vi "D-VASim (Dynamic Virtual Analyzer and Simulator).vi"() -> ()   [LabVIEW 2014]
doc: "D-VASim: Dynamic Virtual Analyzer and Simulator\n\nCreated by Hasan Baig (haba@dtu.dk) at Technical University of Denmark (DTU).s"
uses:
  <vilib>/Utility/miscctls.llb/LVRangeTypeDef.ctl
  <vilib>/Simulation/Implementation/Shared/SIM Continuous Solvers.ctl
  <vilib>/Analysis/Matrix/Datatypes/RealMatrix.ctl
  Sim_Results/SubVIs/Model Information.ctl
  <vilib>/Utility/miscctls.llb/LVPositionTypeDef.ctl
  <vilib>/Utility/error.llb/DialogType.ctl
  Sim_Results/SubVIs/Path.ctl
  <vilib>/Utility/file.llb/Write To Spreadsheet File (string).vi
  <vilib>/Analysis/Matrix/NI_Matrix.lvlib
  <vilib>/Utility/miscctls.llb/LVPointTypeDef.ctl
  <vilib>/Utility/miscctls.llb/LVBoundsTypeDef.ctl
panel:
  out "SBML Components":string
  out "Fn Arg Cnt":string[](array[string])
  out "Comp IDs":string[](array[string])
  out "New Total Pr IDs":string[](array[string])
  out "Math-w/-ch-VarID":string[](array[string])
  out "LP-Cnt_4_Reac":string[](array[string])
  out "Top 3":i32
  out "Top 2":i32
  out "Top 1":i32
  out "Position 10":T1
  out "Position 6":T1
  out "Position 5":T1
  out "Position 4":T1
  out "Left 3":i32
  out "Left 2":i32
  out "Left 1":i32
  out "Position 9":T1
  out "Position 8":T1
  out "Position 7":T1
  out "Position 3":T1
  out "Position 2":T1
  out "Position":T1
  in  "Mod Range":T2={"Minimum"=0.0, "Maximum"=100.0, "Increment"=1.0, "Minor Increment"=1.0, "Start"=0.0}
  in  "Mod_Dimension":u32=62
  out "OnlySubstanceUnits":string[](array[string])
  out "Bound Cond":string[](array[string])
  in  "Final Time":dbl=100.0
  in  "Initial Time":dbl
  in  "ODE Simulation Parameters":T4={"Time Step"=0.1, "Absolute Tolerance"=0.001, "Relative Tolerance"=1e-06, "Continuous Solver"=enum."Adams-Moulton (variable)", "Discrete Time Step"=2.0, "Minimum Time Step"=1e-06, "Maximum Time Step"=1.0, "Initial Time Step"=0.01} {"Initial Time Step" min=0.0; "Maximum Time Step" min=0.0; "Minimum Time Step" min=0.0; "Discrete Time Step" min=0.0; "Relative Tolerance" min=0.0; "Absolute Tolerance" min=0.0; "Time Step" min=0.0}
  out "Pr_Value":string[](array[string])
  out "Pr_Name":string[](array[string])
  out "Pr_Id_Arr":string[](array[string])
  out "Sp_Init_Amnt":string[](array[string])
  out "Sp_Id_Arr":string[](array[string])
  out "Sp_Name":string[](array[string])
  out "Rest_Sp_IDs":string[](array[string])
  out "Rest_Sp_Init_Amnt":string[](array[string])
  out "Rest_Sp_IDs+Names":string[](array[string])
  out "Delta Matrix":T5
  out "Reactant Matrix":T5
  out "Idx of Mod in Sp IDs":i32[](array[numeric])
  out "Out_Tot_Param":string[](array[string])
  out "Out_X_for_ODE":string[](array[string])
  out "Ex_Mod_Init_Amnt":string[](array[string])
  in  "Obtain parameters from Cello UCF":bool
  out "Model Information":T6
  in  "Select SBML Model (.xml)":path
  in  "Generate ODE VI":bool
  in  "Generate SSA VI":bool
  out "Init Sp State (N)":i32[](array[numeric])
  out "Nxt Sp State (N)":i32[](array[numeric])
  out "Equations":string[](array[string])
  out "Sp_for_ODE+Names(X)":string[](array[string])
  out "SP-for-ODE(X)":string[](array[string])
  out "Ex_Mod_IDs":string[](array[string])
  out "ODE File Name":string
  out "ODE VI Name":string
  out "SSA FileName":string
  in  "Tab Control":T7(tab)
  out "Species Info":string[][](table)
  out "Total Species":i32
  out "Parameter info":string[][](table)
  out "Total Parameters":i32
  out "Ordinary Differential Equations":string[][](table)
  out "Reaction Info":string[][](table)
  out "Reaction Math":string[][](table)
  out "Total Reactions":i32
  out "Event Info":string[][](table)
  out "Total Events":i32
  out "Functions Definition":string[][](table)
  out "Total Function Definitions":i32
  out "Units Definition":string[][](table)
  out "Total Units Definitions":i32
  out "Compartments Definition":string[][](table)
  out "Total Compartments":i32
  out "Total Initial Assignments":i32
  out "Initial Assignment":string[][](table)
  out "Rules":string[][](table)
  out "Total Rules":i32
  out "Total Constraints":i32
  out "Constraints":string[][](table)
  out "SSA VI Name":string
  out "Model Folder":path
  out "standard output":string
  out "LP_Values":string[](array[string])
  out "Reactants_Arr":string[](array[string])
  out "Modifiers_Arr":string[](array[string])
  out "LP_IDs":string[](array[string])
  out "Products_Arr":string[](array[string])
  out "R-Stoich":string[](array[string])
  out "P-Stoich":string[](array[string])
  out "Local Parameter Info":string[][](array[string])
  out "standard error":string
  out "Model Name":string
  out "All Param Names":string[](array[string])
  out "All Param Values":string[](array[string])
  out "Init Sp State (S)":string[](array[string])
  out "Nxt Sp State (S)":string[](array[string])
  out "Out_ODE":string[](array[string])
  out "Total Param_IDs":string[](array[string])
  out "Math Expressions":string[](array[string])
  out "SP_for_ODE_Init_Amnt(X)":string[](array[string])
  out "reference Graph":refnum<vi>
  out "Ex_Mod_List":string[](array[string]) caption="Out_List"
  # "D-VASim: Dynamic Virtual Analyzer and Simulator"
  # "Technical University of Denmark"
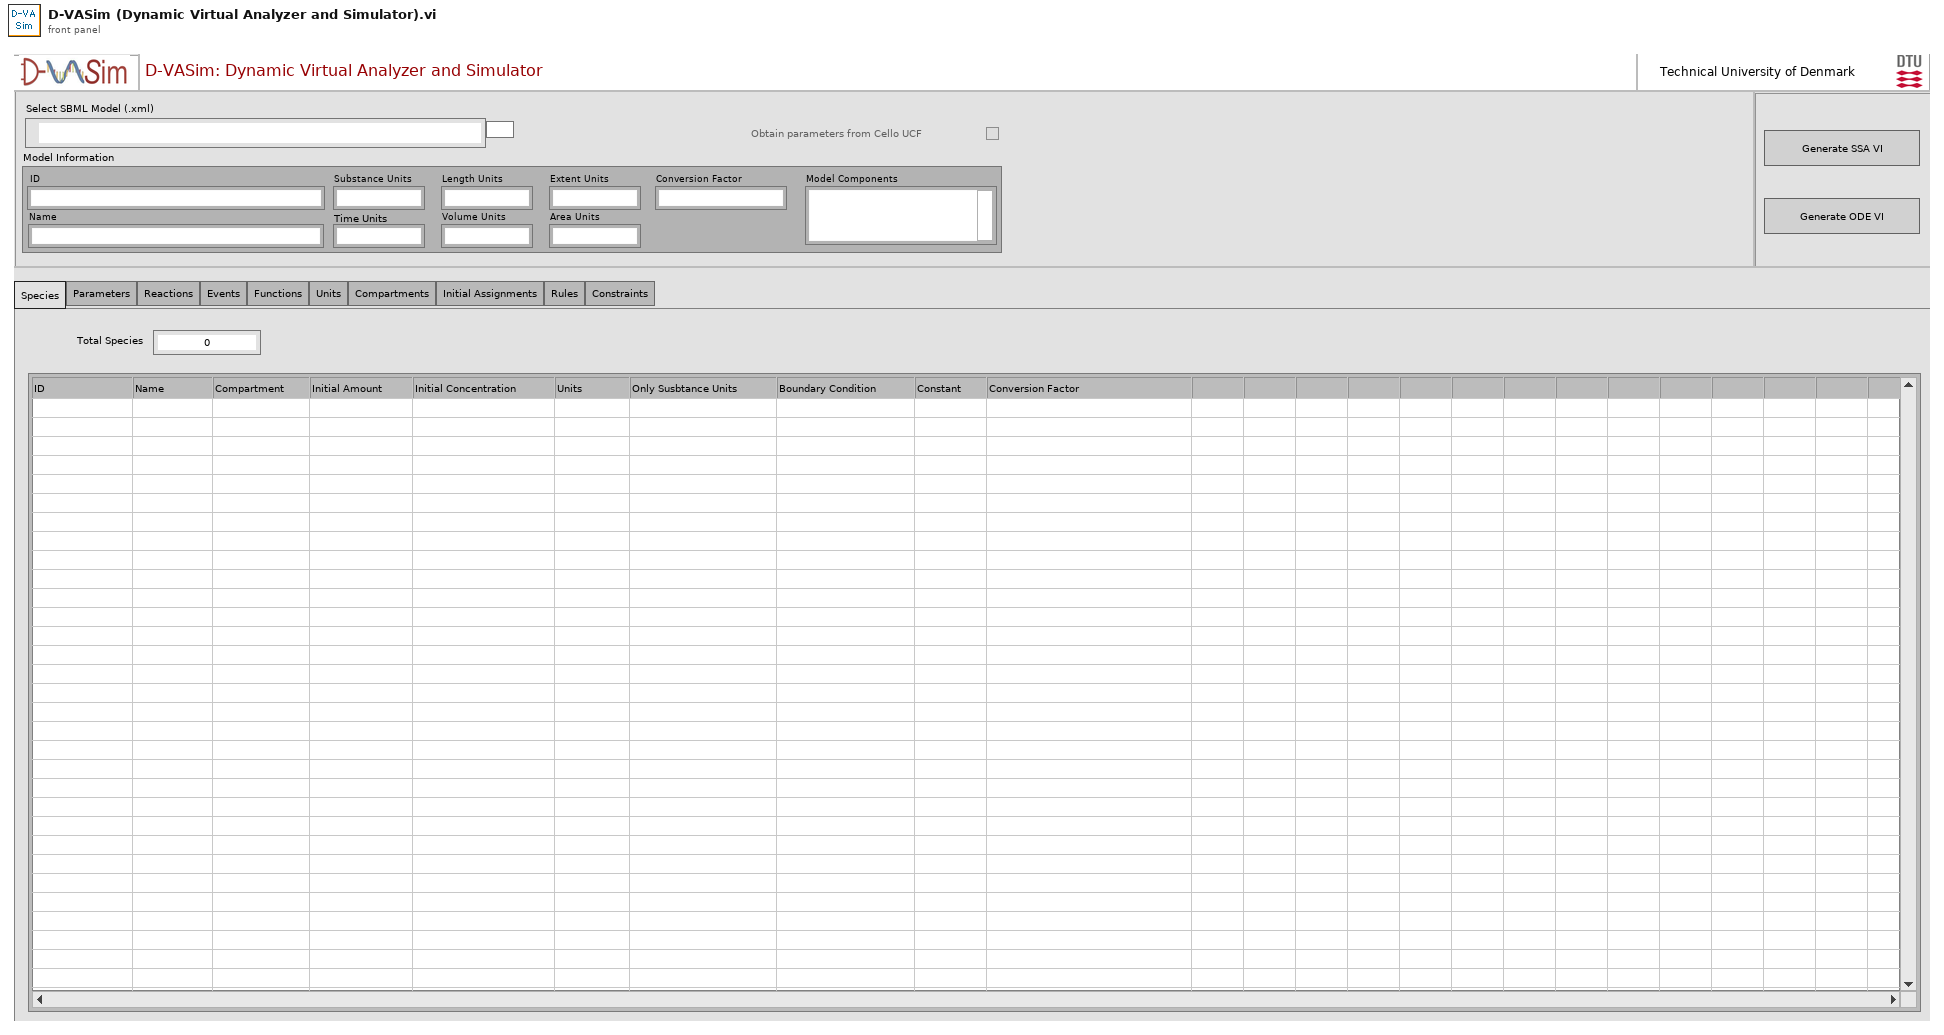
[diagram p1: front panel]
types:
  T1 = typedef "LVPositionTypeDef.ctl" = cluster{"Left":i32, "Top":i32}
  T2 = typedef "LVRangeTypeDef.ctl" = cluster{"Minimum":dbl, "Maximum":dbl, "Increment":dbl, "Minor Increment":dbl, "Start":dbl}
  T3 = typedef "SIM Continuous Solvers.ctl" = enum16{"Runge-Kutta 1 (Euler)", "Runge-Kutta 2", "Runge-Kutta 3", "Runge-Kutta 4", "Runge-Kutta 23 (variable)", "Runge-Kutta 45 (variable)", "BDF (variable)", "Adams-Moulton (variable)", "Rosenbrock (variable)", "Discrete States Only"}
  T4 = cluster{"Time Step":dbl, "Absolute Tolerance":dbl, "Relative Tolerance":dbl, "Continuous Solver":T3, "Discrete Time Step":dbl, "Minimum Time Step":dbl, "Maximum Time Step":dbl, "Initial Time Step":dbl}
  T5 = typedef "NI_Matrix.lvlib/RealMatrix.ctl" = dbl[][]
  T6 = typedef "Model Information.ctl" = cluster{"ID":string, "Name":string, "Substance Units":string, "Time Units":string, "Volume Units":string, "Area Units":string, "Length Units":string, "Extent Units":string, "Conversion Factor":string, "Model Components":string}
  T7 = enum32{"Species", "Parameters", "Reactions", "Events", "Functions", "Units", "Compartments", "Initial Assignments", "Rules", "Constraints"}
  T8 = typedef "DialogType.ctl" = u16
  T9 = typedef "Path.ctl" = string
  T10 = enum32{"Invalid", "Standard", "Closed", "Hidden", "Minimized", "Maximized"}
  T11 = typedef "LVBoundsTypeDef.ctl" = cluster{"Width":u32, "Height":u32}
  T12 = typedef "LVPointTypeDef.ctl" = cluster{"Horizontal":i16, "Vertical":i16}
  T13 = enum32{"invalid app kind", "Development System", "Run Time System", "Student Edition", "Embedded LabVIEW", "Evaluation", "Custom"}
  T14 = cluster{"Model Info":T6, "SpCnt":i32, "Species Info":string[][], "Pr_Cnt":i32, "Parameter info":string[][], "ReacCnt":i32, "Reaction Info":string[][], "Math Expressions":string[][], "EventsCnt":i32, "Event Info":string[][], "UnitsDefCnt":i32, "Units Def":string[][], "CompCnt":i32, "Comp Def":string[][], "Mod_ID":string[], "Mod_Idx":i32[], "RulesCnt":i32, "Rules":string[][], "FuncCnt":i32, "Functions":string[][], "InitAssign Cnt":i32, "Init Assigns":string[][], "ConstraintsCnt":i32, "Constraints":string[][], "Fn Arg Cnt":string[]}
  T15 = cluster{"Reactants_Arr":string[], "R-Stoich":string[], "Products_Arr":string[], "Math Expressions":string[], "P-Stoich":string[], "Bound Cond":string[], "Sp_Id_Arr":string[], "Math-w/-ch-VarID":string[], "OnlySubstanceUnits":string[], "Comp IDs":string[]}
  T16 = cluster{"SP-for-ODE":string[], "Modifiers_Arr":string[], "Sp_Id_Arr":string[], "Sp_Name":string[], "Sp_Init_Amnt":string[], "Reactants_Arr":string[], "Products_Arr":string[]}
  T17 = cluster{"Ex_Mod_IDs":string[], "Ex_Mod_IDs+Names":string[], "Ex_Mod_Init_Amnt":string[], "Rest_Sp_IDs ":string[], "Rest_Sp_IDs+Names":string[], "Rest_Sp_Init_Amnt":string[], "SP_for_ODE_Init_Amnt":string[], "Sp_for_ODE+Names":string[]}
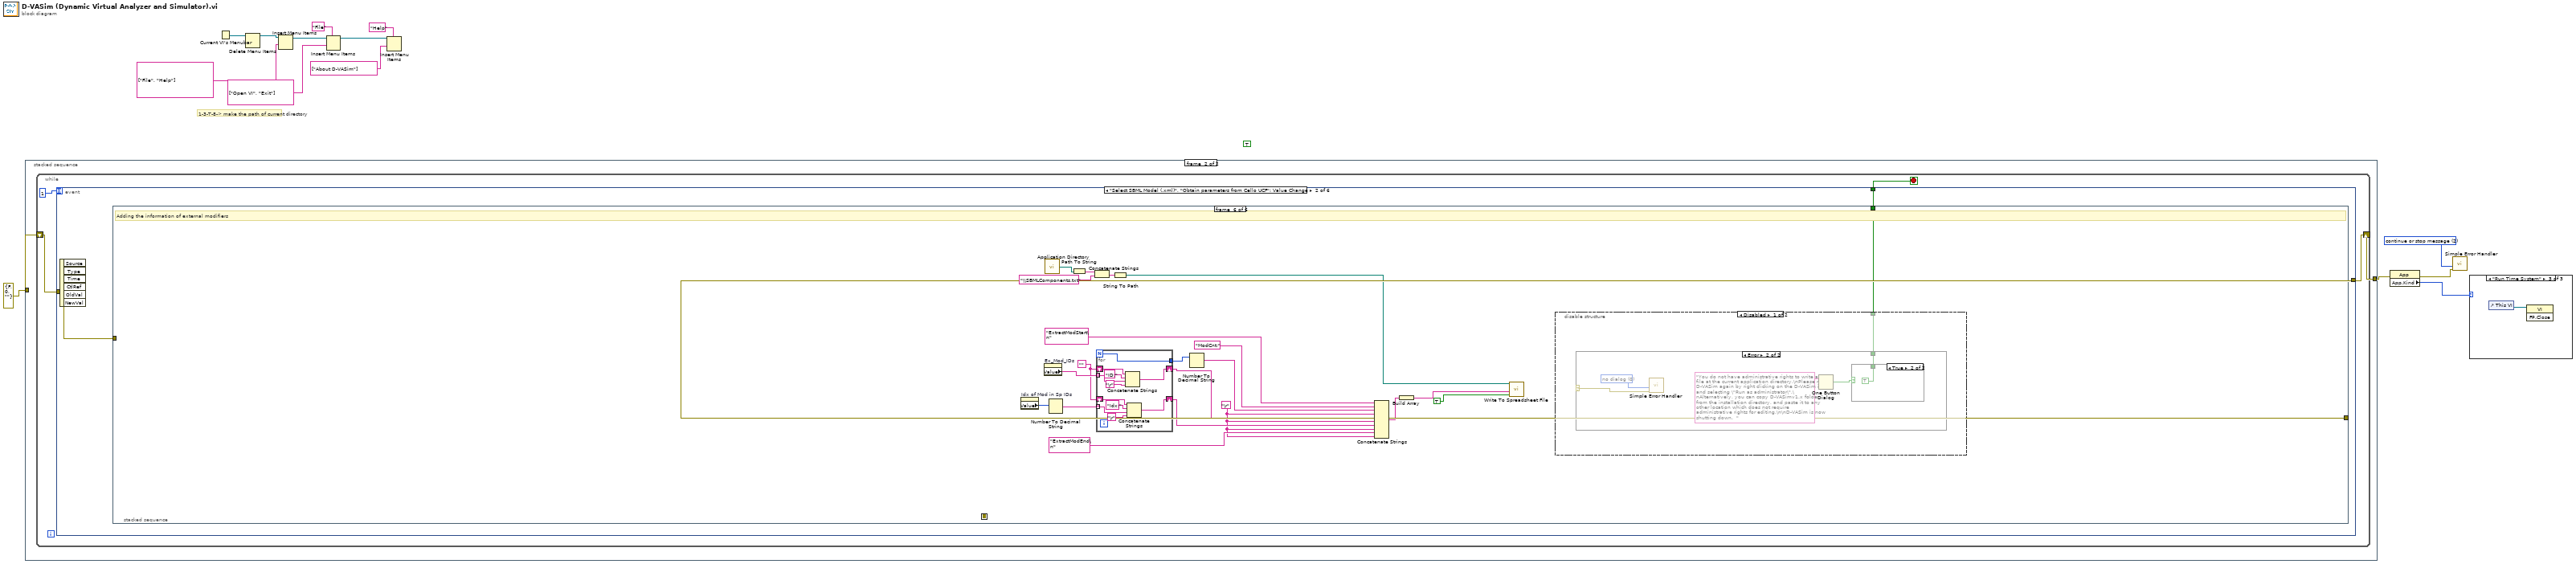
[diagram p0: block diagram]
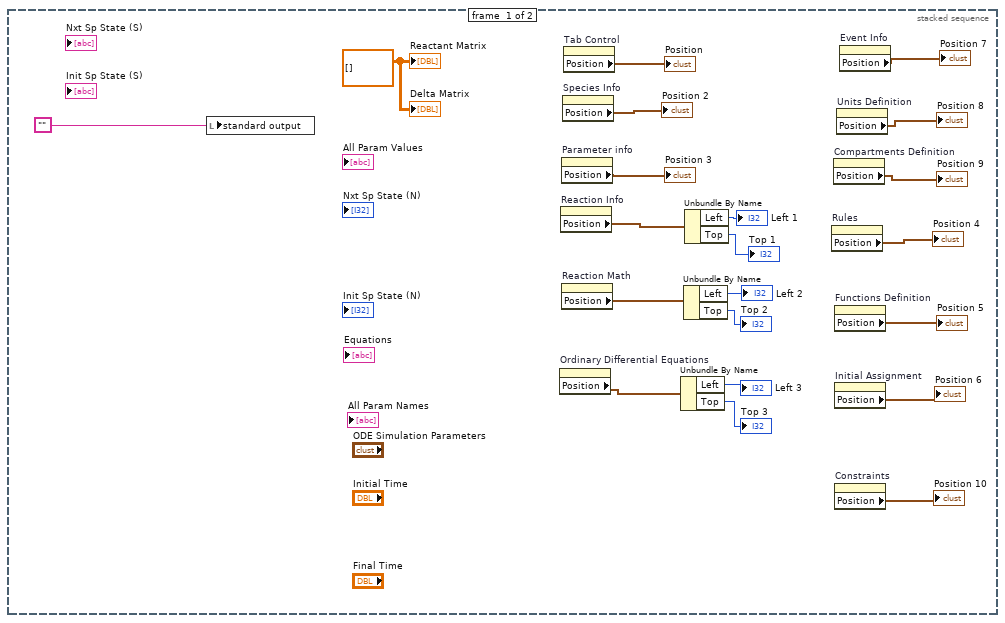
[diagram p4: hidden frame]
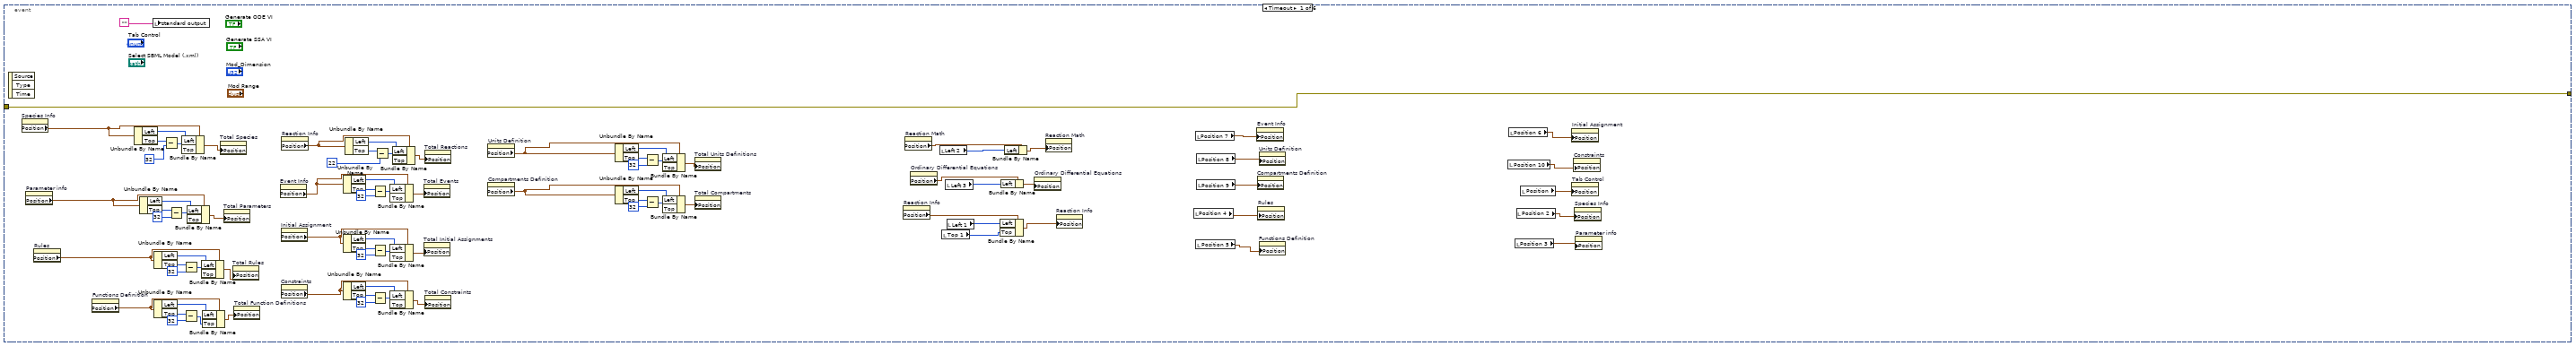
[diagram p5: hidden frame]
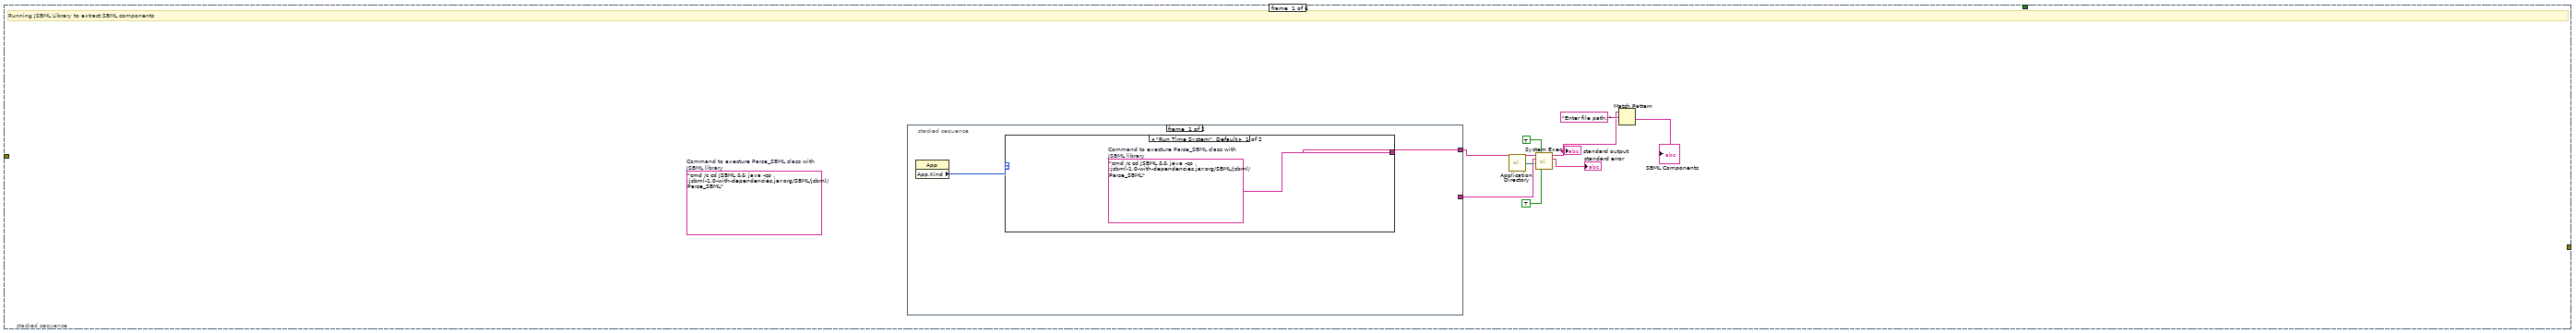
[diagram p6: hidden frame]
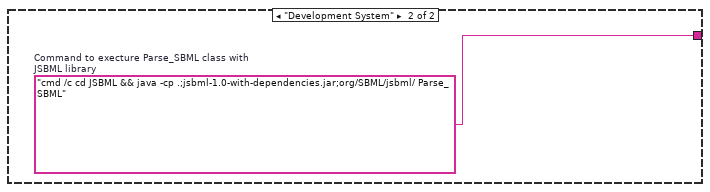
[diagram p7: hidden frame]
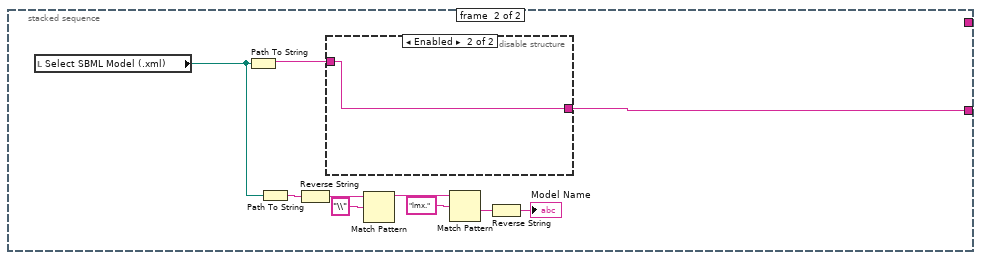
[diagram p8: hidden frame]
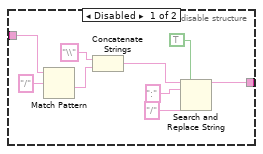
[diagram p9: hidden frame]
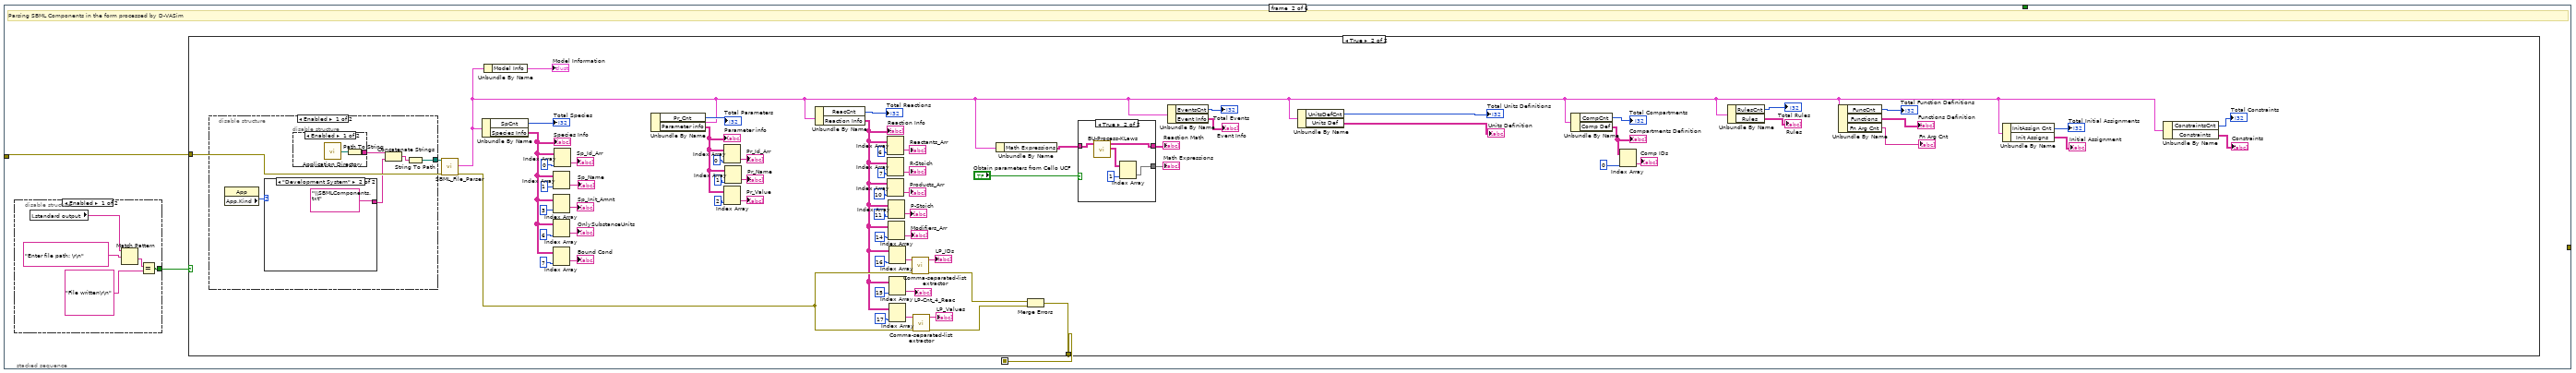
[diagram p10: hidden frame]
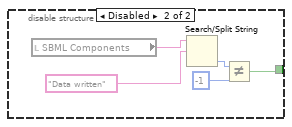
[diagram p11: hidden frame]
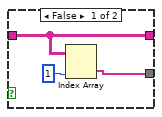
[diagram p13: hidden frame]
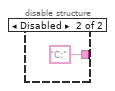
[diagram p14: hidden frame]
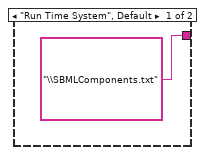
[diagram p15: hidden frame]
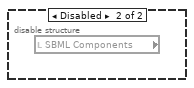
[diagram p16: hidden frame]
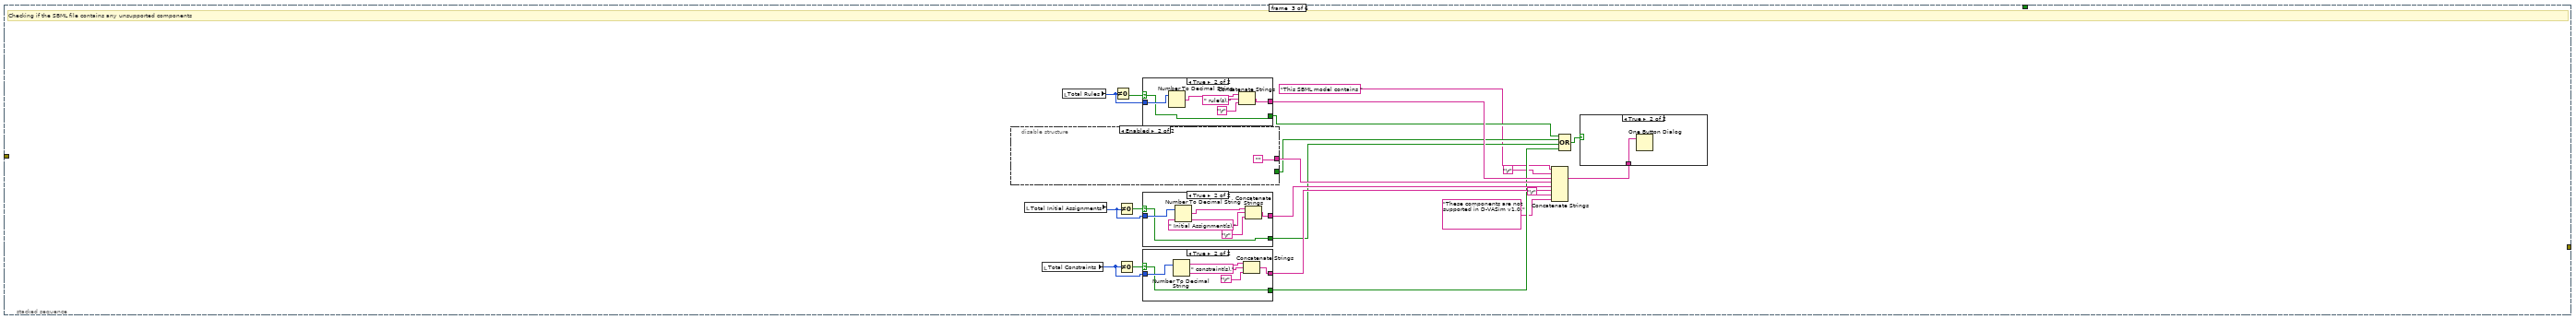
[diagram p17: hidden frame]
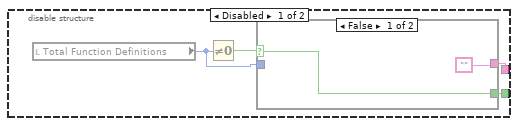
[diagram p18: hidden frame]
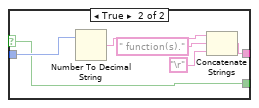
[diagram p19: hidden frame]
diagram:
  (unwired) TRUE ("run minimized? (F)")
  w12 = T8 2 items=["no dialog", "OK message", "continue or stop message", "OK message + warnings", "continue/stop + warnings"] ("type of dialog (OK msg:1)")
  # "1-3-T-8-> make the path of current directory"
  n1 = stacked-sequence {
    tunnel: errorcluster {"status"=FALSE, "code"=0, "source"=""} ("error in (no error)") -> [_ w37]
    tunnel: [_ w36] -> w11
    frame #0 {
      w35 = T5 [] ("Reactant Matrix")
      n2 = local write "standard output"("" ("standard output")) -> ()
      n3 = property on="Ordinary Differential Equations" class="Tbl (strict)"() -> ("Position"=w26:T1)  [unwired: 2 in, 2 out]
      n4 = property on="Reaction Info" class="Tbl (strict)"() -> ("Position"=w25:T1)  [unwired: 2 in, 2 out]
      n5 = property on="Parameter info" class="Tbl (strict)"() -> ("Position"=→"Position 3":T1)  [unwired: 2 in, 2 out]
      n6 = property on="Reaction Math" class="Tbl (strict)"() -> ("Position"=w27:T1)  [unwired: 2 in, 2 out]
      n7 = property on="Species Info" class="Tbl (strict)"() -> ("Position"=→"Position 2":T1)  [unwired: 2 in, 2 out]
      n8 = property on="Tab Control" class="TabCtl (strict)"() -> ("Position"=→"Position":T1)  [unwired: 2 in, 2 out]
      n9 = Unbundle By Name(w26) -> ("Left"=→"Left 3":i32, "Top"=→"Top 3":i32)
      n10 = Unbundle By Name(w27) -> ("Left"=→"Left 2":i32, "Top"=→"Top 2":i32)
      n11 = Unbundle By Name(w25) -> ("Left"=→"Left 1":i32, "Top"=→"Top 1":i32)
      n12 = property on="Rules" class="Tbl (strict)"() -> ("Position"=→"Position 4":T1)  [unwired: 2 in, 2 out]
      n13 = property on="Compartments Definition" class="Tbl (strict)"() -> ("Position"=→"Position 9":T1)  [unwired: 2 in, 2 out]
      n14 = property on="Functions Definition" class="Tbl (strict)"() -> ("Position"=→"Position 5":T1)  [unwired: 2 in, 2 out]
      n15 = property on="Initial Assignment" class="Tbl (strict)"() -> ("Position"=→"Position 6":T1)  [unwired: 2 in, 2 out]
      n16 = property on="Constraints" class="Tbl (strict)"() -> ("Position"=→"Position 10":T1)  [unwired: 2 in, 2 out]
      n17 = property on="Units Definition" class="Tbl (strict)"() -> ("Position"=→"Position 8":T1)  [unwired: 2 in, 2 out]
      n18 = property on="Event Info" class="Tbl (strict)"() -> ("Position"=→"Position 7":T1)  [unwired: 2 in, 2 out]
      "Delta Matrix" <- w35
      "Reactant Matrix" <- w35
    }
    frame #1 {
      n19 = while {
        shift-right: [w39] -> w36
        shift-left: w37 -> [w40]
        stop <- w38 stop-if-true
        n20 = event shown="[1] \"Select SBML Model (.xml)\", \"Obtain parameters from Cello UCF\": Value Change" {
          selector: _ -> [_ _ _ _ _ _]
          dyn-events: _ -> [_ _ _ _ _ _]
          timeout: 1 -> [_ _ _ _ _ _]
          tunnel: w40 -> [w123 w126 w418 w519 w555 _]
          tunnel: [w123 w125 w417 w520 w554 _] -> w39
          tunnel: [_ w124 _ w521 _ TRUE ("NewVal")] -> w38
          event Timeout {
            n21 = event-data() -> ()  [unwired: 1 in, 3 out]
            n22 = property on="Species Info" class="Tbl (strict)"() -> ("Position"=w116:T1)  [unwired: 2 in, 2 out]
            n23 = property on="Parameter info" class="Tbl (strict)"() -> ("Position"=w111:T1)  [unwired: 2 in, 2 out]
            n24 = property on="Rules" class="Tbl (strict)"() -> ("Position"=w71:T1)  [unwired: 2 in, 2 out]
            n25 = property on="Functions Definition" class="Tbl (strict)"() -> ("Position"=w66:T1)  [unwired: 2 in, 2 out]
            n26 = Unbundle By Name(w116) -> ("Left"=w119:i32, "Top"=w121:i32)
            n27 = Unbundle By Name(w111) -> ("Left"=w114:i32, "Top"=w112:i32)
            n28 = local write "standard output"("" ("standard output")) -> ()
            n29 = Unbundle By Name(w71) -> ("Left"=w74:i32, "Top"=w76:i32)
            n30 = Unbundle By Name(w66) -> ("Left"=w69:i32, "Top"=w67:i32)
            n31 = Subtract(x=w121, y=32) -> (x-y=w118:i32)
            n32 = Subtract(x=w112, y=32) -> (x-y=w115:i32)
            n33 = Bundle By Name(cluster=w116, "Left"=w119, "Top"=w118) -> (w117:T1)
            n34 = Subtract(x=w76, y=32) -> (x-y=w73:i32)
            n35 = Subtract(x=w67, y=32) -> (x-y=w70:i32)
            n36 = Bundle By Name(cluster=w111, "Left"=w114, "Top"=w115) -> (w110:T1)
            n37 = Bundle By Name(cluster=w71, "Left"=w74, "Top"=w73) -> (w72:T1)
            n38 = Bundle By Name(cluster=w66, "Left"=w69, "Top"=w70) -> (w65:T1)
            n39 = property on="Total Species" class="DigNum (strict)"("Position"=w117) -> ()  [unwired: 2 in, 2 out]
            n40 = property on="Total Parameters" class="DigNum (strict)"("Position"=w110) -> ()  [unwired: 2 in, 2 out]
            n41 = property on="Total Rules" class="DigNum (strict)"("Position"=w72) -> ()  [unwired: 2 in, 2 out]
            n42 = property on="Total Function Definitions" class="DigNum (strict)"("Position"=w65) -> ()  [unwired: 2 in, 2 out]
            n43 = property on="Event Info" class="Tbl (strict)"() -> ("Position"=w105:T1)  [unwired: 2 in, 2 out]
            n44 = property on="Initial Assignment" class="Tbl (strict)"() -> ("Position"=w60:T1)  [unwired: 2 in, 2 out]
            n45 = property on="Constraints" class="Tbl (strict)"() -> ("Position"=w53:T1)  [unwired: 2 in, 2 out]
            n46 = property on="Reaction Info" class="Tbl (strict)"() -> ("Position"=w45:T1)  [unwired: 2 in, 2 out]
            n47 = Unbundle By Name(w105) -> ("Left"=w108:i32, "Top"=w106:i32)
            n48 = Unbundle By Name(w60) -> ("Left"=w62:i32, "Top"=w64:i32)
            n49 = Unbundle By Name(w53) -> ("Left"=w57:i32, "Top"=w55:i32)
            n50 = Unbundle By Name(w45) -> ("Left"=w47:i32, "Top"=w49:i32)
            n51 = Subtract(x=w106, y=32) -> (x-y=w109:i32)
            n52 = Subtract(x=w64, y=32) -> (x-y=w61:i32)
            n53 = Subtract(x=w55, y=32) -> (x-y=w58:i32)
            n54 = Subtract(x=w49, y=22) -> (x-y=w46:i32)
            n55 = Bundle By Name(cluster=w105, "Left"=w108, "Top"=w109) -> (w104:T1)
            n56 = Bundle By Name(cluster=w60, "Left"=w62, "Top"=w61) -> (w59:T1)
            n57 = Bundle By Name(cluster=w53, "Left"=w57, "Top"=w58) -> (w54:T1)
            n58 = Bundle By Name(cluster=w45, "Left"=w47, "Top"=w46) -> (w44:T1)
            n59 = property on="Total Events" class="DigNum (strict)"("Position"=w104) -> ()  [unwired: 2 in, 2 out]
            n60 = property on="Total Initial Assignments" class="DigNum (strict)"("Position"=w59) -> ()  [unwired: 2 in, 2 out]
            n61 = property on="Total Reactions" class="DigNum (strict)"("Position"=w44) -> ()  [unwired: 2 in, 2 out]
            n62 = property on="Total Constraints" class="DigNum (strict)"("Position"=w54) -> ()  [unwired: 2 in, 2 out]
            n63 = property on="Units Definition" class="Tbl (strict)"() -> ("Position"=w99:T1)  [unwired: 2 in, 2 out]
            n64 = property on="Compartments Definition" class="Tbl (strict)"() -> ("Position"=w93:T1)  [unwired: 2 in, 2 out]
            n65 = Unbundle By Name(w99) -> ("Left"=w101:i32, "Top"=w103:i32)
            n66 = Unbundle By Name(w93) -> ("Left"=w96:i32, "Top"=w94:i32)
            n67 = Subtract(x=w103, y=32) -> (x-y=w100:i32)
            n68 = Subtract(x=w94, y=32) -> (x-y=w97:i32)
            n69 = Bundle By Name(cluster=w99, "Left"=w101, "Top"=w100) -> (w98:T1)
            n70 = Bundle By Name(cluster=w93, "Left"=w96, "Top"=w97) -> (w92:T1)
            n71 = property on="Total Units Definitions" class="DigNum (strict)"("Position"=w98) -> ()  [unwired: 2 in, 2 out]
            n72 = property on="Total Compartments" class="DigNum (strict)"("Position"=w92) -> ()  [unwired: 2 in, 2 out]
            n73 = property on="Reaction Info" class="Tbl (strict)"() -> ("Position"=w43:T1)  [unwired: 2 in, 2 out]
            n74 = property on="Reaction Math" class="Tbl (strict)"() -> ("Position"=w82:T1)  [unwired: 2 in, 2 out]
            n75 = property on="Ordinary Differential Equations" class="Tbl (strict)"() -> ("Position"=w79:T1)  [unwired: 2 in, 2 out]
            n76 = local read "Left 2"() -> (w83:i32)
            n77 = local read "Top 1"() -> (w42:i32)
            n78 = local read "Left 3"() -> (w80:i32)
            n79 = local read "Left 1"() -> (w85:i32)
            n80 = Bundle By Name(cluster=w43, "Left"=w85, "Top"=w42) -> (w84:T1)
            n81 = Bundle By Name(cluster=w79, "Left"=w80) -> (w78:T1)
            n82 = Bundle By Name(cluster=w82, "Left"=w83) -> (w81:T1)
            n83 = property on="Ordinary Differential Equations" class="Tbl (strict)"("Position"=w78) -> ()  [unwired: 2 in, 2 out]
            n84 = property on="Reaction Math" class="Tbl (strict)"("Position"=w81) -> ()  [unwired: 2 in, 2 out]
            n85 = property on="Reaction Info" class="Tbl (strict)"("Position"=w84) -> ()  [unwired: 2 in, 2 out]
            n86 = local read "Position 4"() -> (w77:T1)
            n87 = local read "Position 7"() -> (w88:T1)
            n88 = local read "Position 5"() -> (w52:T1)
            n89 = local read "Position 8"() -> (w87:T1)
            n90 = local read "Position 9"() -> (w86:T1)
            n91 = property on="Event Info" class="Tbl (strict)"("Position"=w88) -> ()  [unwired: 2 in, 2 out]
            n92 = property on="Compartments Definition" class="Tbl (strict)"("Position"=w86) -> ()  [unwired: 2 in, 2 out]
            n93 = property on="Rules" class="Tbl (strict)"("Position"=w77) -> ()  [unwired: 2 in, 2 out]
            n94 = property on="Units Definition" class="Tbl (strict)"("Position"=w87) -> ()  [unwired: 2 in, 2 out]
            n95 = property on="Functions Definition" class="Tbl (strict)"("Position"=w52) -> ()  [unwired: 2 in, 2 out]
            n96 = local read "Position 10"() -> (w50:T1)
            n97 = local read "Position 6"() -> (w51:T1)
            n98 = local read "Position 3"() -> (w89:T1)
            n99 = local read "Position 2"() -> (w90:T1)
            n100 = local read "Position"() -> (w91:T1)
            n101 = property on="Initial Assignment" class="Tbl (strict)"("Position"=w51) -> ()  [unwired: 2 in, 2 out]
            n102 = property on="Tab Control" class="TabCtl (strict)"("Position"=w91) -> ()  [unwired: 2 in, 2 out]
            n103 = property on="Constraints" class="Tbl (strict)"("Position"=w50) -> ()  [unwired: 2 in, 2 out]
            n104 = property on="Species Info" class="Tbl (strict)"("Position"=w90) -> ()  [unwired: 2 in, 2 out]
            n105 = property on="Parameter info" class="Tbl (strict)"("Position"=w89) -> ()  [unwired: 2 in, 2 out]
          }
          event "Select SBML Model (.xml)", "Obtain parameters from Cello UCF": Value Change {
            n106 = event-data() -> ()  [unwired: 1 in, 6 out]
            n107 = stacked-sequence {
              seq-local: [_ w161 _ _ _ _] -> [_ _ _ _ w347 _]
              tunnel: w126 -> [_ w162 _ _ _ _]
              tunnel: [_ _ _ _ w348 _] -> w125
              tunnel: [_ _ _ _ _ w378] -> w124
              frame #0 {
                (unwired) "cmd /c cd JSBML && java -cp .;jsbml-1.0-with-dependencies.jar;org/SBML/jsbml/ Parse_SBML"  # Command to execture Parse_SBML class with JSBML library
                # "Running JSBML Library to extract SBML components"
                n108 = stacked-sequence {
                  tunnel: [w136 _] -> w134
                  tunnel: [_ w140] -> w132
                  frame #0 {
                    n109 = property class="App"() -> ("App.Kind"=w137:T13)  [unwired: 2 in, 2 out]
                    n110 = case shown="\"Run Time System\", Default" w137 {
                      tunnel: [w138 w139] -> w136
                      frame "Run Time System", Default {
                        w138 = "cmd /c cd JSBML && java -cp .;jsbml-1.0-with-dependencies.jar;org/SBML/jsbml/ Parse_SBML"  # Command to execture Parse_SBML class with JSBML library
                      }
                      frame "Development System" {
                        w139 = "cmd /c cd JSBML && java -cp .;jsbml-1.0-with-dependencies.jar;org/SBML/jsbml/ Parse_SBML"  # Command to execture Parse_SBML class with JSBML library
                      }
                    }
                  }
                  frame #1 {
                    n111 = local read "Select SBML Model (.xml)"() -> (w149:path)
                    n112 = Path To String(path=w149) -> (string=w141:string)
                    n113 = Path To String(path=w149) -> (string=w148:string)
                    n114 = Reverse String(1:w148) -> (0:w145:string)
                    n115 = disable-structure shown="Enabled" {
                      disable-tunnel: w141 -> [w154 w159]
                      disable-tunnel: [w150 w159] -> w140
                      frame Disabled {
                        n116 = Match Pattern(string=w154, regular expression="/") -> (after substring=w152:string)  [unwired: 1 in, 3 out]
                        n117 = Concatenate Strings("\\", w152) -> (w151:string)
                        n118 = Search and Replace String(replace all?=TRUE ("replace all? (F)"), input string=w151, search string=":", replace string="/" ("replace string (\"\")")) -> (result string=w150:string)  [unwired: 4 in, 3 out]
                      }
                      frame Enabled {
                      }
                    }
                    n119 = Match Pattern(string=w145, regular expression="\\") -> (before substring=w144:string)  [unwired: 1 in, 3 out]
                    n120 = Match Pattern(string=w144, regular expression="lmx.") -> (after substring=w146:string)  [unwired: 1 in, 3 out]
                    n121 = Reverse String(1:w146) -> (0:→"Model Name":string)
                  }
                }
                n122 = call <vilib>:"Application Directory.vi"() -> ("Application Directory"=w130:path)
                n123 = call <vilib>:"System Exec.vi"("run minimized? (F)"=TRUE, "wait until completion? (T)"=TRUE, "working directory"=w130, "standard input"=w132, "command line"=w134) -> ("standard error"=→"standard error":string, "standard output"=w128:string)  [unwired: 3 in, 2 out]
                "standard output" <- w128
                n124 = Match Pattern(string=w128, regular expression="Enter file path: ") -> (after substring=→"SBML Components":string)  [unwired: 1 in, 3 out]
              }
              frame #1 {
                # "Parsing SBML Components in the form processed by D-VASim"
                n125 = disable-structure shown="Enabled" {
                  disable-tunnel: [w163 w168] -> w160
                  frame Enabled {
                    n126 = local read "standard output"() -> (w167:string)
                    n127 = Match Pattern(string=w167, regular expression="Enter file path: \r\n") -> (after substring=w165:string)  [unwired: 1 in, 3 out]
                    n128 = Equal?(x=w165, y="File written\r\n") -> (x = y?=w163:bool)
                  }
                  frame Disabled {
                    n129 = local read "SBML Components"() -> (w171:string)
                    n130 = Search/Split String(string=w171, search string/char (-)="Data written") -> (offset of match=w170:i32)  [unwired: 1 in, 2 out]
                    n131 = Not Equal?(x=w170, y=-1) -> (x != y?=w168:bool)
                  }
                }
                n132 = case shown="True" w160 {
                  tunnel: w162 -> [w173 w228]
                  tunnel: [w173 w225] -> w161
                  frame False {
                  }
                  frame True {
                    n133 = disable-structure shown="Enabled" {
                      disable-tunnel: [w253 _] -> w224
                      frame Enabled {
                        n134 = property class="App"() -> ("App.Kind"=w252:T13)  [unwired: 2 in, 2 out]
                        n135 = case shown="\"Development System\"" w252 {
                          tunnel: ["\\SBMLComponents.txt" ("string") "\\SBMLComponents.txt" ("string")] -> w251
                          frame "Run Time System", Default {
                          }
                          frame "Development System" {
                          }
                        }
                        n136 = disable-structure shown="Enabled" {
                          disable-tunnel: [w257 "C:"] -> w255
                          frame Enabled {
                            n137 = call <vilib>:"Application Directory.vi"() -> ("Application Directory"=w256:path)
                            n138 = Path To String(path=w256) -> (string=w257:string)
                          }
                          frame Disabled {
                          }
                        }
                        n139 = Concatenate Strings(w255, w251) -> (w254:string)
                        n140 = String To Path(string=w254) -> (path=w253:path)
                      }
                      frame Disabled {
                        n141 = local read "SBML Components"() -> (w261:string)
                      }
                    }
                    n142 = call "SBML_File_Parser.vi"("SBML File"=w224, "error in (no error)"=w228) -> ("SBML Data"=w187:T14, "error out"=w201:errorcluster)  [unwired: 16 in]
                    n143 = Unbundle By Name(w187) -> ("SpCnt"=→"Total Species":i32, "Species Info"=w184:string[][])
                    "Species Info" <- w184
                    n144 = Unbundle By Name(w187) -> ("Model Info"=→"Model Information":T6)
                    n145 = Index Array(array=w184, index (col)=3 ("disabled index (col)")) -> (element=→"Sp_Init_Amnt":string[])  [unwired: 1 in]
                    n146 = Index Array(array=w184, index (col)=6 ("disabled index (col)")) -> (element=→"OnlySubstanceUnits":string[])  [unwired: 1 in]
                    n147 = Index Array(array=w184, index (col)=7 ("disabled index (col)")) -> (element=→"Bound Cond":string[])  [unwired: 1 in]
                    n148 = Index Array(array=w184, index (col)=1 ("disabled index (col)")) -> (element=→"Sp_Name":string[])  [unwired: 1 in]
                    n149 = Index Array(array=w184, index (col)=0 ("disabled index (col)")) -> (element=→"Sp_Id_Arr":string[])  [unwired: 1 in]
                    n150 = Unbundle By Name(w187) -> ("Pr_Cnt"=→"Total Parameters":i32, "Parameter info"=w217:string[][])
                    "Parameter info" <- w217
                    n151 = Index Array(array=w217, index (col)=0 ("disabled index (col)")) -> (element=→"Pr_Id_Arr":string[])  [unwired: 1 in]
                    n152 = Index Array(array=w217, index (col)=2 ("disabled index (col)")) -> (element=→"Pr_Value":string[])  [unwired: 1 in]
                    n153 = Index Array(array=w217, index (col)=1 ("disabled index (col)")) -> (element=→"Pr_Name":string[])  [unwired: 1 in]
                    n154 = Unbundle By Name(w187) -> ("ReacCnt"=→"Total Reactions":i32, "Reaction Info"=w188:string[][])
                    "Reaction Info" <- w188
                    n155 = Index Array(array=w188, index (col)=6 ("disabled index (col)")) -> (element=→"Reactants_Arr":string[])  [unwired: 1 in]
                    n156 = Index Array(array=w188, index (col)=7 ("disabled index (col)")) -> (element=→"R-Stoich":string[])  [unwired: 1 in]
                    n157 = Index Array(array=w188, index (col)=10 ("disabled index (col)")) -> (element=→"Products_Arr":string[])  [unwired: 1 in]
                    n158 = Index Array(array=w188, index (col)=11 ("disabled index (col)")) -> (element=→"P-Stoich":string[])  [unwired: 1 in]
                    n159 = Index Array(array=w188, index (col)=14 ("disabled index (col)")) -> (element=→"Modifiers_Arr":string[])  [unwired: 1 in]
                    n160 = Index Array(array=w188, index (col)=16 ("disabled index (col)")) -> (element=w208:string[])  [unwired: 1 in]
                    n161 = Index Array(array=w188, index (col)=15 ("disabled index (col)")) -> (element=→"LP-Cnt_4_Reac":string[])  [unwired: 1 in]
                    n162 = Index Array(array=w188, index (col)=17 ("disabled index (col)")) -> (element=w207:string[])  [unwired: 1 in]
                    n163 = call "Comma-separated-list extractor.vi"("error in (no error)"=w201, "In_list"=w208) -> ("error out"=w227:errorcluster, "List_Out"=→"LP_IDs":string[])  [unwired: 5 in]
                    n164 = call "Comma-separated-list extractor.vi"("error in (no error)"=w201, "In_list"=w207) -> ("error out"=w226:errorcluster, "List_Out"=→"LP_Values":string[])  [unwired: 5 in]
                    n165 = Unbundle By Name(w187) -> ("Math Expressions"=w206:string[][])
                    n166 = Merge Errors(w227, w226) -> (w225:errorcluster)
                    n167 = case shown="True" "Obtain parameters from Cello UCF" {
                      tunnel: w206 -> [w243 w248]
                      tunnel: [w244 w246] -> w205
                      tunnel: [w243 w247] -> w175
                      frame False {
                        n168 = Index Array(array=w243, index (col)=1 ("disabled index (col)")) -> (element=w244:string[])  [unwired: 1 in]
                      }
                      frame True {
                        n169 = call "BU-Process-KLaws.vi"("Original Set of equations"=w248) -> ("Output Equations w param"=w250:string[][], "Output Equations"=w247:string[][])  [unwired: 9 in]
                        n170 = Index Array(array=w250, index (col)=1 ("disabled index (col)")) -> (element=w246:string[])  [unwired: 1 in]
                      }
                    }
                    "Math Expressions" <- w205
                    "Reaction Math" <- w175
                    n171 = Unbundle By Name(w187) -> ("EventsCnt"=→"Total Events":i32, "Event Info"=→"Event Info":string[][])
                    n172 = Unbundle By Name(w187) -> ("UnitsDefCnt"=→"Total Units Definitions":i32, "Units Def"=→"Units Definition":string[][])
                    n173 = Unbundle By Name(w187) -> ("CompCnt"=→"Total Compartments":i32, "Comp Def"=w181:string[][])
                    "Compartments Definition" <- w181
                    n174 = Index Array(array=w181, index (col)=0 ("disabled index (col)")) -> (element=→"Comp IDs":string[])  [unwired: 1 in]
                    n175 = Unbundle By Name(w187) -> ("RulesCnt"=→"Total Rules":i32, "Rules"=→"Rules":string[][])
                    n176 = Unbundle By Name(w187) -> ("FuncCnt"=→"Total Function Definitions":i32, "Functions"=→"Functions Definition":string[][], "Fn Arg Cnt"=→"Fn Arg Cnt":string[])
                    n177 = Unbundle By Name(w187) -> ("InitAssign Cnt"=→"Total Initial Assignments":i32, "Init Assigns"=→"Initial Assignment":string[][])
                    n178 = Unbundle By Name(w187) -> ("ConstraintsCnt"=→"Total Constraints":i32, "Constraints"=→"Constraints":string[][])
                  }
                }
              }
              frame #2 {
                # "Checking if the SBML file contains any unsupported components"
                n179 = disable-structure shown="Enabled" {
                  disable-tunnel: [w283 ""] -> w274
                  disable-tunnel: [w282 _] -> w269
                  frame Disabled {
                    n180 = local read "Total Function Definitions"() -> (w284:i32)
                    n181 = Not Equal To 0?(x=w284) -> (x != 0?=w285:bool)
                    n182 = case shown="False" w285 {
                      selector: w285 -> [w286 w289]
                      tunnel: w284 -> [_ w293]
                      tunnel: ["" w290] -> w283
                      tunnel: [w286 w289] -> w282
                      frame False {
                      }
                      frame True {
                        n183 = Number To Decimal String(number=w293) -> (decimal integer string=w292:string)  [unwired: 1 in]
                        n184 = Concatenate Strings(w292, " function(s)." ("string"), "\r") -> (w290:string)
                      }
                    }
                  }
                  frame Enabled {
                  }
                }
                n185 = local read "Total Initial Assignments"() -> (w278:i32)
                n186 = local read "Total Constraints"() -> (w276:i32)
                n187 = local read "Total Rules"() -> (w280:i32)
                n188 = Not Equal To 0?(x=w280) -> (x != 0?=w281:bool)
                n189 = Not Equal To 0?(x=w278) -> (x != 0?=w279:bool)
                n190 = Not Equal To 0?(x=w276) -> (x != 0?=w277:bool)
                n191 = case shown="True" w281 {
                  selector: w281 -> [w312 w315]
                  tunnel: w280 -> [_ w319]
                  tunnel: ["" w316] -> w275
                  tunnel: [w312 w315] -> w270
                  frame False {
                  }
                  frame True {
                    n192 = Number To Decimal String(number=w319) -> (decimal integer string=w318:string)  [unwired: 1 in]
                    n193 = Concatenate Strings(w318, " rule(s)." ("string"), "\r") -> (w316:string)
                  }
                }
                n194 = case shown="True" w279 {
                  selector: w279 -> [w304 w307]
                  tunnel: w278 -> [_ w311]
                  tunnel: ["" w308] -> w273
                  tunnel: [w304 w307] -> w268
                  frame False {
                  }
                  frame True {
                    n195 = Number To Decimal String(number=w311) -> (decimal integer string=w310:string)  [unwired: 1 in]
                    n196 = Concatenate Strings(w310, " Initial Assignment(s)." ("string"), "\r") -> (w308:string)
                  }
                }
                n197 = case shown="True" w277 {
                  selector: w277 -> [w296 w299]
                  tunnel: w276 -> [_ w303]
                  tunnel: ["" w300] -> w272
                  tunnel: [w296 w299] -> w267
                  frame False {
                  }
                  frame True {
                    n198 = Number To Decimal String(number=w303) -> (decimal integer string=w302:string)  [unwired: 1 in]
                    n199 = Concatenate Strings(w302, " constraint(s)." ("string"), "\r") -> (w300:string)
                  }
                }
                n200 = Concatenate Strings("This SBML model contains ", "\r", w275, w274, w273, w272, "\r", "These components are not supported in D-VASim v1.0." ("string")) -> (w271:string)
                n201 = Compound Arithmetic op=OR(w270, w269, w268, w267) -> (w266:bool)
                n202 = case shown="True" w266 {
                  tunnel: w271 -> [_ w295]
                  frame False {
                  }
                  frame True {
                    n203 = One Button Dialog(message=w295) -> ()  [unwired: 1 in, 1 out]
                  }
                }
              }
              frame #3 {
                n204 = local read "Math Expressions"() -> (w322:string[])
                n205 = local read "LP-Cnt_4_Reac"() -> (w324:string[])
                n206 = local read "LP_Values"() -> (w332:string[])
                n207 = local read "Sp_Id_Arr"() -> (w326:string[])
                n208 = local read "Pr_Id_Arr"() -> (w325:string[])
                n209 = local read "LP_IDs"() -> (w323:string[])
                n210 = local read "LP_IDs"() -> (w333:string[])
                n211 = local read "Pr_Id_Arr"() -> (w329:string[])
                n212 = local read "LP_IDs"() -> (w330:string[])
                n213 = Build Array(w333, w332) -> (w331:string[][])
                n214 = call "Math-updater-w--for-same-SpVar-names-03022016.vi"("Sp_Id_Arr"=w326, "Math Expressions"=w322, "Pr_Id_Arr"=w325, "LP-Cnt_4_Reac"=w324, "LP_IDs"=w323) -> ("New Total Pr IDs"=→"New Total Pr IDs":string[], "Math-w/-ch-VarID"=→"Math-w/-ch-VarID":string[])
                n215 = Insert Into Array(array=w329, new element=w330) -> (→"Total Param_IDs":string[])  [unwired: 1 in]
                n216 = Transpose 2D Array(2D array=w331) -> (transposed array=→"Local Parameter Info":string[][])
              }
              frame #4 {
                n217 = local read "OnlySubstanceUnits"() -> (w335:string[])
                n218 = local read "Math-w/-ch-VarID"() -> (w338:string[])
                n219 = local read "Math Expressions"() -> (w363:string[])
                n220 = local read "Reactants_Arr"() -> (w366:string[])
                n221 = local read "Products_Arr"() -> (w364:string[])
                n222 = local read "Bound Cond"() -> (w340:string[])
                n223 = local read "Comp IDs"() -> (w334:string[])
                n224 = local read "Sp_Id_Arr"() -> (w339:string[])
                n225 = local read "R-Stoich"() -> (w365:string[])
                n226 = local read "P-Stoich"() -> (w362:string[])
                n227 = Bundle("Reactants_Arr"=w366, "R-Stoich"=w365, "Products_Arr"=w364, "Math Expressions"=w363, "P-Stoich"=w362, "Bound Cond"=w340, "Sp_Id_Arr"=w339, "Math-w/-ch-VarID"=w338, "OnlySubstanceUnits"=w335, "Comp IDs"=w334) -> (w361:T15)  [unwired: 1 in]
                n228 = call "ODE-Generator.vi"("error in (no error)"=w347, "Cluster"=w361) -> ("error out"=w345:errorcluster, "Final ODE 2"=w337:string[], "Final ODE"=w343:string[], "SP-for-ODE"=w346:string[])  [unwired: 4 in]
                "SP-for-ODE(X)" <- w346
                n229 = local read "Reactants_Arr"() -> (w368:string[])
                n230 = local read "Modifiers_Arr"() -> (w372:string[])
                n231 = local read "Sp_Init_Amnt"() -> (w369:string[])
                n232 = local read "Products_Arr"() -> (w367:string[])
                n233 = local read "New Total Pr IDs"() -> (w336:string[])
                n234 = local read "Sp_Id_Arr"() -> (w371:string[])
                n235 = local read "Sp_Name"() -> (w370:string[])
                n236 = Build Array(w343) -> (w342:string[][])
                n237 = Transpose 2D Array(2D array=w342) -> (transposed array=→"Ordinary Differential Equations":string[][])
                n238 = Bundle("SP-for-ODE"=w346, "Modifiers_Arr"=w372, "Sp_Id_Arr"=w371, "Sp_Name"=w370, "Sp_Init_Amnt"=w369, "Reactants_Arr"=w368, "Products_Arr"=w367) -> (w360:T16)  [unwired: 1 in]
                n239 = call "Var-Name-Manipulator-for-ODE-plots.vi"("error in (no error)"=w345, "In_ODE"=w337, "In_Tot_Param"=w336, "In_X_for_ODE"=w346) -> ("error out"=w350:errorcluster, "Out_ODE"=→"Out_ODE":string[], "Out_Tot_Param"=→"Out_Tot_Param":string[], "Out_X_for_ODE"=→"Out_X_for_ODE":string[])  [unwired: 4 in]
                n240 = call "Revised-List_Extractor-Mar31.vi"("Input Cluster"=w360, "error in (no error)"=w345) -> ("Output Cluster"=w359:T17, "error out"=w351:errorcluster)  [unwired: 12 in]
                n241 = Unbundle By Name(w359) -> ("Ex_Mod_IDs"=w344:string[], "Ex_Mod_IDs+Names"=→"Ex_Mod_List":string[], "Ex_Mod_Init_Amnt"=→"Ex_Mod_Init_Amnt":string[], "Rest_Sp_IDs"=→"Rest_Sp_IDs":string[], "Rest_Sp_IDs+Names"=→"Rest_Sp_IDs+Names":string[], "Rest_Sp_Init_Amnt"=→"Rest_Sp_Init_Amnt":string[], "SP_for_ODE_Init_Amnt"=→"SP_for_ODE_Init_Amnt(X)":string[], "Sp_for_ODE+Names"=→"Sp_for_ODE+Names(X)":string[])
                "Ex_Mod_IDs" <- w344
                n242 = local read "Sp_Id_Arr"() -> (w374:string[])
                n243 = call "Index of Mods in Sp ID Array.vi"("error in (no error)"=w351, "Sp_Id_Arr"=w374, "Ex_Mod_IDs"=w344) -> ("error out"=w349:errorcluster, "Idx of Mod in Sp IDs"=→"Idx of Mod in Sp IDs":i32[])  [unwired: 7 in]
                n244 = Merge Errors(w350, w349) -> (w348:errorcluster)
              }
              frame #5 {
                w385 = ""
                w379 = "\r"
                # "Adding the information of external modifiers"
                n245 = property on="Idx of Mod in Sp IDs" class="Arr (strict)"() -> ("Value"=w388:i32[])  [unwired: 2 in, 2 out]
                n246 = property on="Ex_Mod_IDs" class="Arr (strict)"() -> ("Value"=w387:string[])  [unwired: 2 in, 2 out]
                n247 = call <vilib>:"Application Directory.vi"() -> ("Application Directory"=w395:path)
                n248 = Number To Decimal String(number=w388) -> (decimal integer string=w386:string[])  [unwired: 1 in]
                n249 = Path To String(path=w395) -> (string=w397:string)
                n250 = Concatenate Strings(w397, T9 "\\SBMLComponents.txt") -> (w398:string)
                n251 = for {
                  N -> [w408]
                  tunnel: w387 -> [w415] mode=indexing
                  shift-right: [w413] -> w384
                  shift-left: w385 -> [w414]
                  tunnel: w386 -> [w411] mode=indexing
                  shift-right: [w409] -> w383
                  shift-left: w385 -> [w410]
                  tunnel: [w408] -> w381
                  n252 = Concatenate Strings(w414, "ID:" ("string"), w415, "\r") -> (w413:string)
                  n253 = Concatenate Strings(w410, "Idx:" ("string"), w411, "\r") -> (w409:string)
                }
                n254 = String To Path(string=w398) -> (path=w394:path)
                n255 = Number To Decimal String(number=w381) -> (decimal integer string=w380:string)  [unwired: 1 in]
                n256 = Concatenate Strings("ExtractModStart\n" ("string"), "ModCnt:" ("string"), w380, w379, w384, w379, w383, w379, "ExtractModEnd\n" ("string"), w379) -> (w390:string)
                n257 = Build Array(w390) -> (w389:string[])
                n258 = call-poly <vilib>:"Write To Spreadsheet File.vi"("append to file? (new file:F)"=TRUE, "1D data"=w389, "file path (dialog if empty)"=w394) -> ()  [unwired: 5 in, 1 out]
                n259 = disable-structure shown="Disabled" {
                  disable-tunnel: [w399 _] -> w378
                  frame Disabled {
                    n260 = case shown="Error" {
                      selector: _ -> [_ w404]
                      tunnel: [_ w400] -> w399
                      frame No Error {
                      }
                      frame Error {
                        w403 = T8 0 items=["no dialog", "OK message", "continue or stop message", "OK message + warnings", "continue/stop + warnings"] ("type of dialog (OK msg:1)")
                        n261 = call <vilib>:"Simple Error Handler.vi"("type of dialog (OK msg:1)"=w403, "error in (no error)"=w404) -> ()  [unwired: 3 in, 5 out]
                        n262 = One Button Dialog(message="You do not have administrative rights to write a file at the current application directory.\nPlease run D-VASim again by right clicking on the D-VASim icon and selecting \"Run as administrator\".\nAlternatively, you can copy D-VASimv1.x folder, from the installation directory, and paste it to any other location which does not require administrative rights for editing.\n\nD-VASim is now shutting down.  ") -> (true=w401:bool)  [unwired: 1 in]
                        n263 = case shown="True" w401 {
                          tunnel: [_ TRUE ("NewVal")] -> w400
                          frame False {
                          }
                          frame True {
                          }
                        }
                      }
                    }
                  }
                  frame Enabled {
                  }
                }
              }
            }
          }
          event "Generate ODE VI": Value Change {
            n264 = event-data() -> ("NewVal"=w419:bool)  [unwired: 1 in, 5 out]
            n265 = disable-structure shown="Enabled" {
              disable-tunnel: w419 -> [w422 _]
              disable-tunnel: w418 -> [w421 _]
              disable-tunnel: [w420 _] -> w417
              frame Enabled {
                n266 = case shown="True" w422 {
                  tunnel: w421 -> [w423 w425]
                  tunnel: [w423 w424] -> w420
                  frame False {
                  }
                  frame True {
                    n267 = stacked-sequence {
                      seq-local: [w426 _ _ _ _] -> [_ w440 _ _ _]
                      seq-local: [_ w439 _ _ _] -> [_ _ _ _ _]
                      tunnel: w425 -> [w427 _ _ w468 _]
                      tunnel: [_ _ _ w467 _] -> w424
                      frame #0 {
                        # "Copying ODE_Template.vi in Sim_Results folder with the model's name."
                        n268 = disable-structure shown="Enabled" {
                          disable-tunnel: [_ w431] -> w426
                          disable-tunnel: w427 -> [_ w430]
                          frame Disabled {
                          }
                          frame Enabled {
                            n269 = local read "Model Name"() -> (w435:string)
                            n270 = Concatenate Strings(w435, "_ODE" ("string"), ".vi" ("string")) -> (w429:string)
                            "ODE VI Name" <- w429
                            n271 = Concatenate Strings("cmd /c COPY Sim_Results\\SubVIs\\ODE_Template.vi Sim_Results\\" ("command line"), w429) -> (w436:string)
                            n272 = call <vilib>:"Application Directory.vi"() -> ("Application Directory"=w432:path)
                            n273 = call <vilib>:"System Exec.vi"("run minimized? (F)"=TRUE, "error in (no error)"=w430, "working directory"=w432, "command line"=w436) -> ("error out"=w431:errorcluster)  [unwired: 4 in, 3 out]
                          }
                        }
                      }
                      frame #1 {
                        # "Copying SBMLComponents.txt with the model's name in Sim_Results folder"
                        n274 = property class="App"() -> ("App.Kind"=w442:T13)  [unwired: 2 in, 2 out]
                        n275 = case shown="\"Run Time System\"" w442 {
                          tunnel: [_ "cmd /c COPY SBMLComponents.txt Sim_Results\\" ("command line") "cmd /c COPY SBMLComponents.txt Sim_Results\\" ("command line")] -> w441
                          frame "invalid app kind", Default {
                          }
                          frame "Development System" {
                          }
                          frame "Run Time System" {
                          }
                        }
                        n276 = local read "Model Name"() -> (w447:string)
                        n277 = Concatenate Strings(w447, "_ODE" ("string"), ".txt" ("string")) -> (w443:string)
                        "ODE File Name" <- w443
                        n278 = Concatenate Strings(w441, w443) -> (w448:string)
                        n279 = call <vilib>:"Application Directory.vi"() -> ("Application Directory"=w444:path)
                        n280 = call <vilib>:"System Exec.vi"("run minimized? (F)"=TRUE, "error in (no error)"=w440, "working directory"=w444, "command line"=w448) -> ("error out"=w439:errorcluster)  [unwired: 4 in, 3 out]
                      }
                      frame #2 {
                        w452 = "\r\n"
                        n281 = local read "ODE File Name"() -> (w457:string)
                        n282 = call <vilib>:"Application Directory.vi"() -> ("Application Directory"=w463:path)
                        n283 = Path To String(path=w463) -> (string=w465:string)
                        n284 = Concatenate Strings(w465, T9 "\\Sim_Results\\", w457) -> (w466:string)
                        n285 = String To Path(string=w466) -> (path=w462:path)
                        n286 = local read "Out_X_for_ODE"() -> (w453:string[])
                        n287 = local read "Out_Tot_Param"() -> (w456:string[])
                        n288 = local read "Ex_Mod_IDs"() -> (w455:string[])
                        n289 = local read "Out_ODE"() -> (w454:string[])
                        n290 = Concatenate Strings("ODE Info----\n" ("string"), w452, w456, w452, w455, w452, w454, w452, w453, w452, "ODE Info ends----\n" ("string")) -> (w459:string)
                        n291 = Build Array(w459) -> (w458:string[])
                        n292 = call-poly <vilib>:"Write To Spreadsheet File.vi"("append to file? (new file:F)"=TRUE, "1D data"=w458, "file path (dialog if empty)"=w462) -> ()  [unwired: 5 in, 1 out]
                      }
                      frame #3 {
                        # "Launching ODE VI of a model"
                        n293 = disable-structure shown="Enabled" {
                          disable-tunnel: [w471 _] -> w467
                          disable-tunnel: w468 -> [w469 _]
                          frame Enabled {
                            n294 = disable-structure shown="Enabled" {
                              disable-tunnel: [w479 w484] -> w476
                              frame Disabled {
                                n295 = local read "Model Folder"() -> (w480:path)
                                n296 = local read "SSA VI Name"() -> (w478:string)
                                n297 = Path To String(path=w480) -> (string=w482:string)
                                n298 = Concatenate Strings(w482, ":", w478) -> (w481:string)
                                n299 = String To Path(string=w481) -> (path=w479:path)
                              }
                              frame Enabled {
                                n300 = local read "ODE VI Name"() -> (w485:string)
                                n301 = call <vilib>:"Application Directory.vi"() -> ("Application Directory"=w486:path)
                                n302 = Path To String(path=w486) -> (string=w488:string)
                                n303 = Concatenate Strings(w488, T9 "\\Sim_Results\\", w485) -> (w489:string)
                                n304 = String To Path(string=w489) -> (path=w484:path)
                              }
                            }
                            n305 = Open VI Reference(vi path=w476, error in (no error)=w469) -> (vi reference=w474:refnum<vi>, error out=w475:errorcluster)  [unwired: 4 in]
                            n306 = invoke class="VI" method="FP.Open"(reference=w474, error in=w475, "State"=T10."Standard") -> (reference out=w473:refnum<vi>, error out=w472:errorcluster)  [unwired: 2 in, 3 out]
                            n307 = invoke class="VI" method="Run VI"(reference=w473, error in=w472, "Wait until done"=FALSE ("Wait Until Done")) -> (error out=w471:errorcluster)  [unwired: 2 in, 4 out]
                          }
                          frame Disabled {
                          }
                        }
                      }
                      frame #4 {
                        # "Creating a graph plot"
                        n308 = disable-structure shown="Disabled" {
                          frame Disabled {
                            n309 = stacked-sequence {
                              frame #0 {
                                n310 = stacked-sequence {
                                seq-local: [w493 _] -> [_ w498]
                                frame #0 {
                                w495 = 21716 items=[".NET Container"=2125, ".NET Refnum"=3441, "2D Picture"=3508, "3D Picture"=23776, "Absolute Value"=1054, "Access Rights"=1412, "ActiveX Container"=2072, "Add"=1050, "Add (with error terminals)"=3915, "Add Array Elements"=1903, "Agitator"=3831, "AllSpoll"=1960, "Always Copy"=2400, "And"=1061, "And Array Elements"=1911, "Append True/False String"=1511, "Application Refnum"=3412, "Array (block diagram constant)"=2070, "Array (classic)"=3300, "Array (modern)"=21608, "Array Interface Control"=23777, "Array Max & Min"=1907, "Array of Strings to Path"=1422, "Array Size"=1809, "Array Subset"=2044, "Array To Cluster"=1168, "Array To Spreadsheet String"=1540, "Atmospheric Tank (classic)"=3070, "Atmospheric Tank (modern)"=21751, "Automation Close"=8001, "Automation Open"=8000, "Automation Refnum"=3410, "Avogadro Constant (1/mol)"=23520, "Base 10 Logarithm Of e"=23512, "Bin #1"=3073, "Bin #2"=21755, "Bitpack to Array"=3135, "Bluetooth Close Connection"=9148, "Bluetooth Create Listener"=9151, "Bluetooth Discover"=9152, "Bluetooth Network Connection Refnum"=3468, "Bluetooth Open Connection"=9153, "Bluetooth Read"=9149, "Bluetooth Wait On Listener"=9147, "Bluetooth Write"=9150, "Boolean Array To Number"=1815, "Boolean To (0,1)"=1167, "Build Array"=2041, "Build Cluster Array"=2047, "Build Matrix"=8500, "Build Path"=1419, "Build Waveform"=2066, "Bundle"=2049, "Bundle By Name"=2057, "Byte Array To String"=1609, "Byte Stream File Refnum"=3408, "Call By Reference"=3901, "Call Chain"=1999, "Call Library Function Node"=2062, "Call Parent Method"=2354, "CAN Channel (block diagram constant)"=2124, "CAN Channel (classic)"=3340, "CAN Channel (modern)"=21817, "CAN Channel (system)"=21966, "CAN Interface (block diagram constant)"=2123, "CAN Interface (classic)"=3339, "CAN Interface (modern)"=21815, "CAN Interface (system)"=21964, "CAN Task (block diagram constant)"=3471, "CAN Task (classic)"=3470, "CAN Task (modern)"=21789, "CAN Task (system)"=21963, "Cancel Button (modern)"=21739, "Cancel Button (system)"=3131, "Cancel Notification"=9107, "Carriage Return Constant"=23500, "Case Structure"=2001, "Cast Unit Bases"=1079, "Check Valve"=3833, "Checkbox (classic)"=3117, "CheckBox (modern)"=21924, "Checkbox (system)"=3132, "Class Specifier Constant"=2094, "Classic Color Box"=3013, "Classic Color Ramp"=3022, "Classic Horizontal Slide Switch"=3114, "Classic Vertical Slide"=3004, "Clear Fixed-Point Overflow Status"=5562, "Close File"=8052, "Close File (deprecated)"=1405, "Close Reference"=8011, "Close Variable Connection"=23783, "Cluster (classic)"=3400, "Cluster (modern)"=21607, "Cluster Constant"=2071, "Cluster To Array"=1169, "Code Interface Node"=2050, "Coerce To Type"=2402, "Color Box Constant"=2120, "Color Box Thin Border"=2905, "Colored Rectangle (broken?)"=3625, "Combo Box (classic)"=3304, "Combo Box (modern)"=21604, "Combo Box (system)"=21917, "Combo Box Constant"=2088, "Complex Conjugate"=1048, "Complex To Polar"=1045, "Complex To Re/Im"=1044, "Compound Arithmetic"=2200, "Compressor"=3832, "Concatenate Strings"=2040, "Conditional Disable Structure"=2064, "Constructor Node"=3904, "Control & Simulation Loop"=2099, "Control Help Window"=1353, "Control Online Help"=1355, "Control Refnum"=3419, "Convert Unit"=2059, "Conveyer"=3827, "Copy"=8053, "Copy (deprecated)"=1416, "Cosecant"=1204, "Cosine"=1201, "Cotangent"=1205, "CPU Information"=24130, "Create Folder"=8055, "Create Network Stream Endpoint"=23793, "Create Network Stream Reader Endpoint"=23811, "Create Network Stream Writer Endpoint"=23810, "Create Stream"=23796, "Create Unique Network Stream Endpoint"=23795, "Create Unique Network Stream Reader Endpoint"=23807, "Create Unique Network Stream Writer Endpoint"=23806, "Create User Event"=2073, "Current Processor ID"=24131, "Current VI's Menubar"=9000, "Current VI's Path"=1426, "DAQmx Analog Trigger Source (block diagram constant)"=2119, "DAQmx Analog Trigger Source (classic)"=3336, "DAQmx Analog Trigger Source (modern)"=21774, "DAQmx Analog Trigger Source (system)"=21951, "DAQmx Device Name (block diagram constant)"=2093, "DAQmx Device Name (classic)"=3318, "DAQmx Device Name (modern)"=21773, "DAQmx Device Name (system)"=21950, "DAQmx Global Channel (block diagram constant)"=3430, "DAQmx Global Channel (classic)"=3443, "DAQmx Global Channel (modern)"=21770, "DAQmx Global Channel (system)"=21957, "DAQmx Physical Channel (block diagram constant)"=2118, "DAQmx Physical Channel (classic)"=3335, "DAQmx Physical Channel (modern)"=21777, "DAQmx Physical Channel (system)"=21954, "DAQmx Scale Name (block diagram constant)"=2116, "DAQmx Scale Name (classic)"=3317, "DAQmx Scale Name (modern)"=21775, "DAQmx Scale Name (system)"=21952, "DAQmx Switch (block diagram constant)"=2121, "DAQmx Switch (classic)"=3337, "DAQmx Switch (modern)"=21776, "DAQmx Switch (system)"=21953, "DAQmx Task Name (block diagram constant)"=3434, "DAQmx Task Name (classic)"=3442, "DAQmx Task Name (modern)"=21778, "DAQmx Task Name (system)"=21959, "DAQmx Terminal (block diagram constant)"=2117, "DAQmx Terminal (classic)"=3319, "DAQmx Terminal (modern)"=21781, "DAQmx Terminal (system)"=21955, "Data Cache Size"=24132, "Data Log File Refnum"=3402, "Data Value Reference"=3476, "Data Value Reference Constant"=24134, "DataSocket Close"=1085, "DataSocket Open"=1084, "DataSocket Read"=1086, "DataSocket Refnum"=3417, "DataSocket Write"=1087, "Date/Time To Seconds"=1308, "Decimal Digit?"=1119, "Decimal String To Number"=1184, "Decimate 1D Array"=2046, "DecomposeArray"=2412, "DecomposeLockDataValRef"=2406, "DecomposeVariant"=2404, "Decrement"=1058, "Default Directory"=1427, "Delete"=8056, "Delete (deprecated)"=1417, "Delete Data Value Reference"=2409, "Delete From Array"=3912, "Delete Menu Items"=9004, "Delete Variant Attribute"=8206, "Delete Waveform Attribute"=8209, "Deny Access"=8057, "Dequeue Element"=9113, "Destroy Stream Endpoint"=23794, "Destroy User Event"=2075, "DevClear"=1961, "DevClearList"=1962, "Device Control/Status"=1433, "Device Refnum"=3405, "Diagram Disable Structure"=2054, "Dial (classic)"=3050, "Dial (modern)"=21732, "Digital Data (classic)"=3210, "Digital Data (modern)"=21216, "Digital Waveform Graph (classic)"=3511, "Digital Waveform Graph (modern)"=21718, "Direct Variable Read"=23785, "Direct Variable Write"=23788, "Divide"=1053, "Divide (with error terminals)"=3918, "Dlg Horiz Scrollbar"=21905, "Dlg Mac Group Box"=32514, "Dlg Numeric #1"=2100, "Dlg Numeric #2"=3006, "Dlg String"=2110, "Dlg Vert Scrollbar"=21906, "Down Arrow"=3824, "Down Bow Valve (flat)"=3707, "Down Bow Valve (outline)"=3807, "Down Bow Valve (shaded)"=21767, "Down Rect Valve (flat)"=3706, "Down Rect Valve (outline)"=3806, "Down Rect Valve (shaded)"=21766, "Down Tee (flat)"=3818, "Down Tee (shaded)"=3718, "Dynamic FPGA Interface Cast"=5690, "Eased Corner Rectangle"=32513, "Elementary Charge (C)"=23517, "Empty Array?"=23063, "Empty Path Constant"=23523, "Empty String Constant"=23503, "Empty String/Path?"=1112, "Enable Menu Tracking"=9002, "EnableLocal"=1963, "EnableRemote"=1964, "End of Line Constant"=23525, "Enqueue Element"=9111, "Enqueue Element At Opposite End"=9129, "Enum (classic)"=3023, "Enum (modern)"=21605, "Enum (system)"=3062, "Enum Constant"=2090, "EOF"=1410, "Equal To 0?"=1113, "Equal?"=1102, "Error Ring Constant"=2039, "Event Callback Refnum"=3435, "Event Data Node"=2102, "Event Structure"=2052, "Exchanger"=3828, "Exclusive Or"=1063, "Exponential"=1211, "Exponential (Arg) -1"=1222, "Expression Node"=2201, "False Constant"=2006, "Feedback Node"=2353, "FieldPoint IO Point (block diagram constant)"=3440, "FieldPoint IO Point (classic)"=3439, "FieldPoint IO Point (modern)"=21784, "FIFO Refnum"=3474, "File Dialog"=8058, "File Dialog (deprecated)"=8081, "File Path Control (classic)"=3203, "File Path Control (modern)"=21730, "File Path Control (system)"=21922, "File Path Indicator (classic)"=3204, "File Path Indicator (modern)"=21731, "File/Directory Info"=8082, "File/Directory Info (deprecated)"=1413, "FindLstn"=1965, "FindRQS"=1966, "First Call?"=1083, "Fixed-Point Overflow?"=5565, "Fixed-Point to Integer Cast"=5566, "Flat Box"=3602, "Flat Circle"=3605, "Flat Down Triangle"=3623, "Flat Frame"=3608, "Flat Left Triangle"=3620, "Flat Right Triangle"=3621, "Flat Round Button"=3102, "Flat Rounded Box"=3611, "Flat Sequence Structure"=2069, "Flat Square Button"=3103, "Flat Up Triangle"=3622, "Flatten To JSON"=24201, "Flatten To String"=1164, "Flatten To XML"=8400, "Flattened String To Variant"=8202, "Floating Point Equal?"=23064, "Flush Event Queue"=2135, "Flush File"=8059, "Flush File (deprecated)"=1406, "Flush Queue"=9114, "Flush Stream"=23808, "For Loop"=2002, "Fork"=2194, "Format Date/Time String"=8100, "Format Into File"=2083, "Format Into String"=2081, "Format Value"=1512, "Formula Node"=2004, "FPGA Refnum to Session"=2322, "Fract/Exp String To Number"=1187, "Framed Color Box (classic)"=3008, "Framed Color Box (modern)"=21019, "Free Label"=2321, "Furnace"=3829, "Gauge (classic)"=3040, "Gauge (modern)"=21009, "Gauge for Simon"=32600, "Generate Front Panel Activity"=1329, "Generate Occurrence"=1700, "Generate User Event"=2074, "Generate User-Defined Trace Event"=2250, "Get Control Values by Index"=24204, "Get Datalog Position"=8061, "Get Date/Time In Seconds"=1303, "Get Date/Time String"=1600, "Get Drag Drop Data"=9154, "Get File Position"=8062, "Get File Size"=8063, "Get Fixed-Point Components"=11163, "Get Help Window Status"=1354, "Get Matrix Diagonal"=8501, "Get Matrix Elements"=8502, "Get Menu Item Info"=9005, "Get Menu Selection"=9001, "Get Menu Short Cut Info"=9007, "Get Notifier Status"=9103, "Get Number of Records"=8064, "Get Permissions"=8065, "Get Queue Status"=9110, "Get Submatrix"=8503, "Get Type and Creator"=8066, "Get Variant Attribute"=8205, "Get Volume Info"=8067, "Get Waveform Attribute"=8208, "Get Waveform Components"=2067, "Global Variable"=2060, "GPIB Clear"=1954, "GPIB Initialization"=1957, "GPIB Misc"=1956, "GPIB Read"=1951, "GPIB Serial Poll"=1955, "GPIB Status"=1959, "GPIB Trigger"=1953, "GPIB Wait"=1958, "GPIB Write"=1950, "Gravitational Constant (N m2/kg2)"=23519, "Greater Or Equal To 0?"=1114, "Greater Or Equal?"=1103, "Greater Than 0?"=1117, "Greater?"=1110, "Handle Peek"=1604, "Handle Poke"=1605, "Hex Digit?"=1123, "Hexadecimal String To Number"=1185, "Hopper #1"=21754, "Hopper #2"=3072, "Horiz Line"=3821, "Horiz Pipe (flat)"=3810, "Horiz Pipe (shaded)"=3710, "Horizontal Button Box"=3636, "Horizontal Fill Slide (classic)"=3012, "Horizontal Fill Slide (modern)"=21100, "Horizontal Gradient Oval"=32502, "Horizontal Gradient Rectangle"=32504, "Horizontal Gradient Rounded Rectangle"=32507, "Horizontal Graduated Bar"=21106, "Horizontal Pointer Slide (classic)"=3011, "Horizontal Pointer Slide (modern)"=21101, "Horizontal Pointer Slide (system)"=21902, "Horizontal Progress Bar (modern)"=21102, "Horizontal Progress Bar (system)"=21910, "Horizontal Scrollbar"=21110, "Horizontal Slide (classic)"=3010, "Horizontal Slide (system)"=21904, "Horizontal Smooth Box"=3633, "Horizontal Splitter Bar"=21861, "Horizontal Splitter Bar (Classic)"=21863, "Horizontal Splitter Bar (System)"=21865, "Horizontal Switch"=3108, "Horizontal Tank"=3071, "Horizontal Toggle Switch (classic)"=3110, "Horizontal Toggle Switch (modern)"=21700, "Hyperbolic Cosecant"=23053, "Hyperbolic Cosine"=1215, "Hyperbolic Cotangent"=23055, "Hyperbolic Secant"=23054, "Hyperbolic Sine"=1214, "Hyperbolic Tangent"=1216, "IMAQ Session"=3415, "Implies"=1080, "In Place Element Structure"=2360, "In Range and Coerce"=1127, "Include Fixed-Point Overflow Status"=5564, "Increment"=1057, "Index & Bundle Cluster Array"=2056, "Index Array"=2042, "Index String Array"=1531, "Initialize Array"=2053, "Inline C Node"=2104, "Insert Into Array"=3911, "Insert Menu Items"=9003, "Integer to Fixed-Point Cast"=5567, "Intensity Chart (classic)"=3509, "Intensity Chart (modern)"=21719, "Intensity Graph (classic)"=3510, "Intensity Graph (modern)"=21720, "Interleave 1D Arrays"=2045, "Interpolate 1D Array"=1905, "Inverse Cosecant"=23050, "Inverse Cosine"=1207, "Inverse Cotangent"=23052, "Inverse Hyperbolic Cosecant"=23056, "Inverse Hyperbolic Cosine"=1218, "Inverse Hyperbolic Cotangent"=23058, "Inverse Hyperbolic Secant"=23057, "Inverse Hyperbolic Sine"=1217, "Inverse Hyperbolic Tangent"=1219, "Inverse Secant"=23051, "Inverse Sine"=1206, "Inverse Tangent"=1208, "Inverse Tangent (2 Input)"=1228, "Invoke Node"=3900, "IP To String"=1710, "IrDA Close Connection"=9144, "IrDA Create Listener"=9140, "IrDA Discover"=9141, "IrDA Network Connection Refnum"=3450, "IrDA Open Connection"=9142, "IrDA Read"=9145, "IrDA Wait On Listener"=9143, "IrDA Write"=9146, "IVI Delete Session"=8103, "IVI Logical Name (block diagram constant)"=3420, "IVI Logical Name (classic)"=3414, "IVI Logical Name (modern)"=21736, "IVI New Session"=8102, "Join"=2195, "Join Numbers"=1171, "Junction"=2197, "Knob (classic)"=3005, "Knob (modern)"=21000, "Label (modern)"=21960, "Label (system)"=21961, "Labeled Oblong Button"=3125, "Labeled Rectangular Button"=3124, "Labeled Round Button"=3122, "Labeled Square Button"=3123, "LabVIEW Object"=3457, "Leak Variant Value Reference"=2410, "LED Button"=3116, "Left Arrow"=3826, "Left Bow Valve (flat)"=3701, "Left Bow Valve (outline)"=3801, "Left Bow Valve (shaded)"=21761, "Left Down Elbow (flat)"=3811, "Left Down Elbow (shaded)"=3711, "Left Pump (flat)"=3813, "Left Pump (shaded)"=3713, "Left Rect Valve (flat)"=3700, "Left Rect Valve (outline)"=3800, "Left Rect Valve (shaded)"=21760, "Left Tee (flat)"=3809, "Left Tee (shaded)"=3709, "Left Up Elbow (flat)"=3808, "Left Up Elbow (shaded)"=3708, "Less Or Equal To 0?"=1115, "Less Or Equal?"=1104, "Less Than 0?"=1118, "Less?"=1111, "Lexical Class"=1126, "Line (chiseled, system)"=3632, "Line (chiseled, thick)"=3630, "Line (chiseled, thin)"=3627, "Line (thick)"=3629, "Line (thin)"=3626, "Line Feed Constant"=23501, "Line with Arrow (thick)"=3631, "Line with Arrow (thin)"=3628, "List Directory"=1418, "List Folder"=8083, "Listbox (classic)"=21806, "Listbox (modern)"=21792, "Listbox (system)"=21805, "Listbox Symbol Ring Constant"=2038, "Local Variable"=2061, "Lock Range"=1411, "Logarithm Base 10"=1210, "Logarithm Base 2"=1225, "Logarithm Base X"=1224, "Logical Shift"=1081, "Lossy Enqueue Element"=9130, "Lowered Box (thick)"=3635, "Lowered Rounded Box"=3638, "Machine Epsilon"=23528, "MakeAddr"=1967, "Mantissa & Exponent"=1150, "Match First String"=1532, "Match Pattern"=1535, "Match True/False String"=1533, "MathScript Call By Reference"=3906, "MathScript Node"=2357, "MATLAB script"=9020, "Matrix Size"=8507, "Max & Min"=1108, "Menu Refnum"=3413, "Menu Ring (classic)"=3018, "Menu Ring (modern)"=21600, "Menu-Popup Ring"=3017, "Merge Errors"=2147, "Merge Signals"=2350, "Meter (classic)"=3030, "Meter (modern)"=21008, "Mixed Checkbox (system)"=21333, "Mixed Signal Graph"=21721, "Molar Gas Constant (J/(mol K))"=23522, "Motion Resource (block diagram constant)"=3449, "Motion Resource (classic)"=3448, "Motion Resource (modern)"=21787, "Motor (flat)"=3820, "Motor (shaded)"=3720, "Move"=8068, "Move (deprecated)"=1415, "Multi-Segment Pipe"=23780, "Multicolumn Listbox (classic)"=21799, "Multicolumn Listbox (modern)"=21791, "Multicolumn Listbox (system)"=21798, "Multiply"=1052, "Multiply (with error terminals)"=3917, "Multiply Array Elements"=1904, "Multirate Structure"=2199, "Natural Logarithm"=1209, "Natural Logarithm (Arg +1)"=1221, "Natural Logarithm Base"=23510, "Natural Logarithm Of 10"=23513, "Natural Logarithm Of 2"=23514, "Natural Logarithm Of Pi"=23508, "Negate"=1069, "Negative Infinity"=23509, "New Data Value Reference"=2408, "New Directory"=1402, "New File"=1404, "New VI"=8014, "New VI Object"=8015, "Not"=1064, "Not A Number/Path/Refnum?"=1128, "Not A Path Constant"=23524, "Not a Refnum Constant"=23526, "Not a Shared Variable"=23527, "Not And"=1071, "Not Equal To 0?"=1116, "Not Equal?"=1105, "Not Exclusive Or"=1073, "Not Or"=1072, "Notifier Refnum"=3423, "Number of Cache Levels"=24133, "Number To Boolean Array"=1814, "Number To Decimal String"=1180, "Number To Engineering String"=1183, "Number To Exponential String"=1505, "Number To Fractional String"=1506, "Number To Hexadecimal String"=1181, "Number To Octal String"=1182, "Numeric Constant"=2005, "Numeric Control (classic)"=3000, "Numeric Control (modern)"=21003, "Numeric Control (system)"=21919, "Numeric Indicator (classic)"=3001, "Numeric Indicator (modern)"=21004, "Obtain Notifier"=9101, "Obtain Queue"=9108, "Occurrence Refnum"=3406, "Octal Digit?"=1129, "Octal String To Number"=1186, "OK Button (modern)"=21738, "OK Button (system)"=3130, "Old VISA Open"=1921, "OLE Variant"=3150, "One Button Dialog"=1340, "Open and Verify Variable Connection"=23790, "Open Application Reference"=8012, "Open Device"=1430, "Open Dynamic Bitfile Reference"=5691, "Open File"=1403, "Open Tank (flat classic)"=21752, "Open Tank (shaded classic)"=3074, "Open Variable Connection"=23779, "Open Variable Connection in Background"=23791, "Open VI Object Reference"=8013, "Open VI Reference"=8010, "Open/Create/Replace Datalog"=8054, "Open/Create/Replace File"=8050, "Or"=1062, "Or Array Elements"=1910, "Oval with Shadow"=32509, "Package Matrix"=23001, "PassControl"=1968, "Path Constant"=2009, "Path to Array of Strings"=1423, "Path To String"=1077, "Path Type"=1421, "Pi"=23504, "Pi Divided By 2"=23506, "Pi Multiplied By 2"=23505, "Pick Line"=1510, "Pict Ring (classic)"=3015, "Pict Ring (modern)"=21602, "Pict Ring (system)"=21925, "PixMap"=3505, "PixMap (warning: dangerous)"=3507, "Planck's Constant (J/Hz)"=23516, "Platform Flat Square Button"=3134, "Plug-In Control"=21820, "Polar To Complex"=1047, "Polar To Re/Im"=23061, "Positive Infinity"=23515, "Power Of 10"=1212, "Power Of 2"=1223, "Power Of X"=1213, "PPoll"=1969, "PPollConfig"=1970, "PPollUnconfig"=1971, "Preallocated Read from Binary File"=24135, "Preserve Run-Time Class"=8018, "Pressure Tank (flat)"=3075, "Pressure Tank (shaded)"=21753, "Preview Queue Element"=9112, "Printable?"=1124, "Property Node"=1920, "Pulldown Menu Ring"=3061, "Push Button"=21001, "Queue Refnum"=3424, "Quit LabVIEW"=1352, "Quotient & Remainder"=1056, "Radio Button (system)"=3133, "Radio Buttons (classic)"=22003, "Radio Buttons (modern)"=22001, "Radio Buttons (system)"=22002, "Raised Box (classic)"=3600, "Raised Box (modern)"=3637, "Raised Circle"=3603, "Raised Down Triangle"=3615, "Raised Frame"=3606, "Raised Left Triangle"=3612, "Raised Right Triangle"=3613, "Raised Rounded Box"=3609, "Raised Up Triangle"=3614, "Random Number (0-1)"=1070, "RcvRespMsg"=1972, "Re/Im To Complex"=1046, "Re/Im To Polar"=23060, "Read Datalog"=8069, "Read Device"=1432, "Read File"=1407, "Read from Binary File"=8051, "Read from Text File"=8070, "Read Multiple Elements from Stream"=23803, "Read Single Element from Stream"=23797, "Read Variable"=23781, "Read Variable with Timeout"=23786, "ReadStatus"=1973, "Receive"=1974, "ReceiveSetup"=1975, "Recessed Box"=3601, "Recessed Circle"=3604, "Recessed Down Triangle"=3619, "Recessed Frame (modern)"=3607, "Recessed Frame (system)"=3624, "Recessed Left Triangle"=3616, "Recessed Menu Ring"=3019, "Recessed Right Triangle"=3617, "Recessed Rounded Box"=3610, "Recessed Up Triangle"=3618, "Reciprocal"=1059, "Reciprocal Of e"=23511, "Reciprocal Of Pi"=23507, "RecomposeArray"=2403, "RecomposeUnlockDataValRef (warning: dangerous)"=2407, "RecomposeVariant (warning: dangerous)"=2405, "Rectangular Stop Button"=3128, "Refnum to Path"=1424, "Refnum to Session"=2306, "Region"=2196, "Register Event Callback"=2078, "Register For Events"=2065, "Register Session"=2319, "Release Notifier"=9102, "Release Queue"=9109, "Remove Fixed-Point Overflow Status"=5563, "Replace Array Subset"=3910, "Replace Substring"=3913, "Request Deallocation"=1610, "ResetSys"=1976, "Reshape Array"=2055, "Resize Matrix"=8508, "Resource Index"=1088, "Reverse 1D Array"=1900, "Reverse String"=1537, "Right Arrow"=3825, "Right Bow Valve (flat)"=3705, "Right Bow Valve (outline)"=3805, "Right Bow Valve (shaded)"=21765, "Right Down Elbow (flat)"=3817, "Right Down Elbow (shaded)"=3717, "Right Pump (flat)"=3819, "Right Pump (shaded)"=3719, "Right Rect Valve (flat)"=3704, "Right Rect Valve (outline)"=3804, "Right Rect Valve (shaded)"=21764, "Right Tee (flat)"=3815, "Right Tee (shaded)"=3715, "Right Up Elbow (flat)"=3814, "Right Up Elbow (shaded)"=3714, "Rocker"=21002, "Rotary Feeder"=3830, "Rotate"=1082, "Rotate 1D Array"=1906, "Rotate Left With Carry"=1606, "Rotate Right With Carry"=1607, "Rotate String"=1536, "Round Button"=3100, "Round LED (classic)"=3120, "Round LED (modern)"=21012, "Round Light"=3104, "Round Push Button"=3118, "Round Push Button (profile)"=3112, "Round Radio Button"=3106, "Round Stop Button"=3127, "Round To Nearest"=1055, "Round Toward +Infinity"=1076, "Round Toward -Infinity"=1075, "Rounded Rectangle with Shadow"=32508, "RT FIFO Create"=24000, "RT FIFO Delete"=24003, "RT FIFO Read"=24001, "RT FIFO Write"=24002, "Rydberg Constant (1/m)"=23521, "Scale By Power Of 2"=1074, "Scan From File"=2082, "Scan From String"=2080, "Scan String For Tokens"=8101, "Scan Value"=1534, "Scanned Variable Read"=23784, "Scanned Variable Write"=23787, "Search 1D Array"=1901, "Search and Replace String"=3914, "Search Variable Container"=23802, "Search/Split String"=1538, "Secant"=1203, "Seconds To Date/Time"=1309, "Seek"=1409, "Select"=1516, "Send"=1977, "Send Notification"=9104, "SendCmds"=1978, "SendDataBytes"=1979, "SendIFC"=1980, "SendList"=1981, "SendLLO"=1982, "SendSetup"=1983, "Session to Refnum"=2307, "Set Control Values by Index"=24203, "Set Datalog Position"=8072, "Set File Position"=8073, "Set File Size"=8074, "Set Matrix Diagonal"=8504, "Set Matrix Elements"=8505, "Set Menu Item Info"=9006, "Set Number of Records"=8075, "Set Occurrence"=1702, "Set Permissions"=8076, "Set Submatrix"=8506, "Set Type and Creator"=8077, "Set Variant Attribute"=8204, "Set Waveform Attribute"=8207, "SetRWLS"=1984, "SetTimeOut"=1985, "Shared Variable"=23778, "Shared Variable Constant"=3473, "Shared Variable Control (classic)"=3472, "Shared Variable Control (modern)"=21814, "Shared Variable to String"=1831, "Sign"=1049, "Simple Horizontal Slide"=3003, "Simple Numeric"=2900, "Simple String"=2115, "Simple Vertical Slide"=3002, "Sinc"=1227, "Sine"=1200, "Sine & Cosine"=1220, "Size Handle"=1603, "Slide Switch"=21011, "Smoothed Oval"=32500, "Smoothed Rounded Rectangle"=32505, "Sort 1D Array"=1120, "Sort Array of String"=23065, "Speed Of Light In Vacuum (m/sec)"=23518, "Spin Control (system)"=21900, "Split 1D Array"=1908, "Split Button"=21020, "Split Number"=1170, "Split Signals"=2351, "Spreadsheet String To Array"=1539, "Square"=23059, "Square Button"=3101, "Square LED (classic)"=3121, "Square LED (modern)"=21013, "Square Light"=3105, "Square Push Button"=3119, "Square Push Button (profile)"=3113, "Square Radio Button"=3107, "Square Root"=1060, "Stacked Sequence Structure"=2000, "State"=2198, "State Diagram"=2051, "Static VI Reference"=2084, "Stop"=1350, "Stop Button"=21230, "String Constant"=2007, "String Control (classic)"=3200, "String Control (modern)"=21701, "String Control (system)"=21920, "String Indicator (classic)"=3201, "String Indicator (modern)"=21702, "String Length"=1502, "String Subset"=1503, "String To Byte Array"=1608, "String To IP"=1711, "String To Path"=1078, "String to Shared Variable"=1830, "Strip Path"=1420, "SubPanel"=21810, "SubPanel (Classic)"=21811, "SubPanel (System)"=21823, "Subtract"=1051, "Subtract (with error terminals)"=3916, "Swap Bytes"=1162, "Swap Values"=2401, "Swap Vector Element"=1912, "Swap Words"=1163, "Tab Constant"=23502, "Tab Control (classic)"=3330, "Tab Control (modern)"=3332, "Tab Control (system)"=3331, "Table (classic)"=21796, "Table (modern)"=21790, "Table (system)"=21797, "Tag Attribute Ring"=2063, "Tangent"=1202, "Tank (classic)"=3020, "Tank (modern)"=21006, "TCP Close Connection"=1713, "TCP Create Listener"=1717, "TCP Flattened Read"=1718, "TCP Flattened Write"=1719, "TCP Flex Read"=1720, "TCP Flex Write"=1721, "TCP Network Connection Refnum"=3407, "TCP Open Connection"=1715, "TCP Read"=1716, "TCP Wait On Listener"=1712, "TCP Write"=1714, "TDMS Advanced Asynchronous Read (Data Ref)"=2151, "TDMS Advanced Asynchronous Write (Data Ref)"=2150, "TDMS Close"=24113, "TDMS Configure Asynchronous Reads (Data Ref)"=2153, "TDMS Configure Asynchronous Writes (Data Ref)"=2152, "TDMS Defragment"=24119, "TDMS File"=3477, "TDMS Flush"=24117, "TDMS Get Asynchronous Read Status (Data Ref)"=2155, "TDMS Get Asynchronous Write Status (Data Ref)"=2154, "TDMS Get Properties"=24115, "TDMS In Memory Close"=2157, "TDMS In Memory Open"=2156, "TDMS In Memory Read Bytes"=2158, "TDMS List Contents"=24116, "TDMS Open"=24112, "TDMS Read"=24111, "TDMS Refnum To File ID"=24120, "TDMS Set Properties"=24114, "TDMS Write"=24110, "TDMS Write IP"=24118, "Temporary Directory"=1435, "TestSRQ"=1986, "TestSys"=1987, "Text & Pict Ring (classic)"=3016, "Text & Pict Ring (modern)"=21603, "Text Button"=21015, "Text Ring (block diagram constant)"=2008, "Text Ring (classic)"=3014, "Text Ring (modern)"=21601, "Text Ring (system)"=3060, "Text to UTF-8"=23066, "Thermometer (classic)"=3021, "Thermometer (modern)"=21007, "Threshold 1D Array"=1909, "Tick Count (ms)"=1300, "Time Stamp (block diagram constant)"=2068, "Time Stamp Control (classic)"=5555, "Time Stamp Control (modern)"=21913, "Time Stamp Control (system)"=21967, "Time Stamp Indicator (classic)"=5556, "Time Stamp Indicator (modern)"=21914, "Timed Loop"=5570, "Timed Sequence"=5573, "To Byte Integer"=1140, "To Double Precision Complex"=1152, "To Double Precision Float"=1147, "To Extended Precision Complex"=1154, "To Extended Precision Float"=1149, "To Fixed-Point"=5561, "To Long Integer"=1142, "To Lower Case"=1189, "To More Generic Class"=8017, "To More Specific Class"=8016, "To OLE Variant"=8002, "To Probe String"=2413, "To Quad Integer"=1155, "To Single Precision Complex"=1151, "To Single Precision Float"=1146, "To Time Stamp"=5560, "To Unsigned Byte Integer"=1143, "To Unsigned Long Integer"=1145, "To Unsigned Quad Integer"=1156, "To Unsigned Word Integer"=1144, "To Upper Case"=1188, "To Variant"=8201, "To Word Integer"=1141, "Traditional DAQ Channel (block diagram constant)"=2085, "Traditional DAQ Channel (classic)"=3320, "Traditional DAQ Channel (modern)"=21733, "Transpose 1D Array"=23068, "Transpose 2D Array"=1902, "Transpose Matrix"=8509, "Tree (classic)"=21819, "Tree (modern)"=21793, "Tree (system)"=21794, "Trigger"=1988, "TriggerList"=1989, "Two Button Dialog"=1341, "Type and Creator"=1434, "Type Cast"=1166, "UDP Close"=1726, "UDP Multicast Open"=1727, "UDP Network Connection Refnum"=3418, "UDP Open"=1723, "UDP Read"=1724, "UDP Write"=1725, "Unbitpack from Array"=3136, "Unbundle"=2048, "Unbundle By Name"=2058, "Unflatten From JSON"=24202, "Unflatten From String"=1165, "Unflatten From XML"=8401, "Unleak Variant Value Reference"=2411, "Unpackage Matrix"=23000, "Unregister For Events"=2076, "Unregister Session"=2320, "Up Arrow"=3823, "Up Bow Valve (flat)"=3703, "Up Bow Valve (outline)"=3803, "Up Bow Valve (shaded)"=21763, "Up Rect Valve (flat)"=3702, "Up Rect Valve (outline)"=21762, "Up Rect Valve (shaded)"=3802, "Up Tee (flat)"=3812, "Up Tee (shaded)"=3712, "User Defined Refnum"=3428, "User Defined Refnum Tag (block diagram constant)"=3426, "User Defined Refnum Tag (classic)"=3429, "User Defined Refnum Tag (modern)"=21745, "User Defined Refnum Tag Flatten (classic)"=3454, "User Defined Refnum Tag Flatten (modern)"=21747, "User Defined Tag (block diagram constant)"=2114, "User Defined Tag (classic)"=3329, "User Defined Tag (modern)"=21749, "User Item"=3506, "UTF-8 to Text"=23067, "Variable Class Specifier Constant"=2106, "Variable Name Constant"=3478, "Variant"=3310, "Variant To Data"=8003, "Variant To Flattened String"=8203, "Vert Line"=3822, "Vert Pipe (flat)"=3816, "Vert Pipe (shaded)"=3716, "Vert Rocker"=21740, "Vertical Fill Slide (classic)"=3009, "Vertical Fill Slide (modern)"=21014, "Vertical Gradient Oval"=32501, "Vertical Gradient Rectangle"=32503, "Vertical Gradient Rounded Rectangle"=32506, "Vertical Graduated Bar"=21107, "Vertical Pointer Slide (classic)"=3007, "Vertical Pointer Slide (modern)"=21017, "Vertical Pointer Slide (system)"=21901, "Vertical Progress Bar (modern)"=21104, "Vertical Progress Bar (system)"=21909, "Vertical Scrollbar"=21111, "Vertical Slide (system)"=21903, "Vertical Slide Switch (classic)"=3115, "Vertical Slide Switch (modern)"=21741, "Vertical Smooth Box"=3634, "Vertical Splitter Bar"=21860, "Vertical Splitter Bar (Classic)"=21862, "Vertical Splitter Bar (System)"=21864, "Vertical Switch"=3109, "Vertical Toggle Switch (classic)"=3111, "Vertical Toggle Switch (modern)"=21005, "VI Library"=1425, "VI Refnum"=3422, "VI Server Reference"=2091, "VISA Assert Interrupt Signal"=2309, "VISA Assert Trigger"=1929, "VISA Assert Utility Signal"=2310, "VISA Clear"=1927, "VISA Close"=1922, "VISA Disable Event"=1940, "VISA Discard Events"=1941, "VISA Enable Event"=1942, "VISA Find Resource"=1923, "VISA Flush I/O Buffer"=2302, "VISA GPIB Command"=2315, "VISA GPIB Control ATN"=2316, "VISA GPIB Control REN"=2304, "VISA GPIB Pass Control"=2317, "VISA GPIB Send IFC"=2318, "VISA In 16"=1930, "VISA In 32"=1944, "VISA In 64"=2140, "VISA In 8"=1936, "VISA Lock"=1993, "VISA Map Address"=1932, "VISA Map Trigger"=2311, "VISA Memory Allocation"=1997, "VISA Memory Allocation Ex"=2146, "VISA Memory Free"=1998, "VISA Move"=2303, "VISA Move In 16"=1948, "VISA Move In 32"=1991, "VISA Move In 64"=2144, "VISA Move In 8"=1946, "VISA Move Out 16"=1949, "VISA Move Out 32"=1992, "VISA Move Out 64"=2145, "VISA Move Out 8"=1947, "VISA Open"=2308, "VISA Out 16"=1931, "VISA Out 32"=1945, "VISA Out 64"=2141, "VISA Out 8"=1937, "VISA Peek 16"=1934, "VISA Peek 32"=1995, "VISA Peek 64"=2142, "VISA Peek 8"=1938, "VISA Poke 16"=1935, "VISA Poke 32"=1996, "VISA Poke 64"=2143, "VISA Poke 8"=1939, "VISA Read"=1925, "VISA Read STB"=1928, "VISA Read To File"=2313, "VISA Refnum to Session"=2300, "VISA Resource Name"=3421, "VISA resource name (classic)"=3409, "VISA resource name (modern)"=21737, "VISA Set I/O Buffer Size"=2301, "VISA Status Description"=1924, "VISA Unlock"=1994, "VISA Unmap Address"=1933, "VISA Unmap Trigger"=2312, "VISA USB Control In"=2086, "VISA USB Control Out"=2087, "VISA VXI Cmd or Query"=2305, "VISA Wait on Event"=1943, "VISA Write"=1926, "VISA Write From File"=2314, "Volume Info"=1414, "Wait (ms)"=1302, "Wait For Activity"=1722, "Wait For Front Panel Activity"=1328, "Wait for GPIB RQS"=1952, "Wait on Notification"=9105, "Wait on Notification from Multiple"=9106, "Wait on Notification from Multiple with Notifier History"=9132, "Wait on Notification with Notifier History"=9131, "Wait on Occurrence"=1701, "Wait Until Next ms Multiple"=1327, "WaitSRQ"=1990, "Waveform Chart"=21010, "Waveform Chart (classic)"=3501, "Waveform Chart (modern)"=21717, "Waveform Graph (classic)"=3504, "Waveform Graph (modern)"=21703, "While Loop #1"=2003, "While Loop #2"=2352, "White Space?"=1125, "Write Datalog"=8079, "Write Device"=1431, "Write File"=1408, "Write Multiple Elements to Stream"=23804, "Write Single Element to Stream"=23798, "Write to Binary File"=8078, "Write to Text File"=8080, "Write Variable"=23782, "Write Variable with Timeout"=23789, "XY Graph (classic)"=3500, "XY Graph (modern)"=21716, "Y-th Root of X"=23062]
                                w497 = refnum<vi> refnum  # XYGraph
                                n311 = local read item#-1() -> ()  [unwired: 1 out]
                                n312 = New VI Object(vi object class=w497, style=w495, position/next to=T12 {"Horizontal"=300, "Vertical"=0} ("location")) -> (object refnum=w490:refnum<vi>)  [unwired: 5 in, 1 out]
                                "reference Graph" <- w490
                                n313 = property class="XYGraph"(reference=w490, "Plot Area Size"=T11 {"Width"=760, "Height"=500} ("Plot Area:Size")) -> (reference out=w492:refnum<vi>, "Terminal"=w493:refnum<vi>)  [unwired: 1 in, 1 out]
                                n314 = property class="XYGraph"(reference=w492, "Terminal.Position"=T1 {"Left"=100, "Top"=100} ("Position")) -> ()  [unwired: 1 in, 2 out]
                                }
                                frame #1 {
                                n315 = local read item#-1() -> (w499)
                                n316 = Index Array(array=w499, index=4) -> (element=w501)
                                n317 = invoke class="CtrlTerm" method="Connect Wire"(reference=w498, "Wire Source"=w501) -> ()  [unwired: 5 in, 7 out]
                                }
                                }
                              }
                              frame #1 {
                                n318 = local read item#-1() -> ()  [unwired: 1 out]
                                n319 = invoke class="VI" method="BD.CleanUp"() -> ()  [unwired: 3 in, 3 out]
                              }
                              frame #2 {
                                n320 = local read "SP-for-ODE(X)"() -> (w504:string[])
                                n321 = local read "reference Graph"() -> (w503:refnum<vi>)
                                n322 = Array Size(array=w504) -> (size(s)=w505:i32)
                                n323 = for {
                                tunnel: w504 -> [w514] mode=indexing
                                tunnel: w503 -> [w518]
                                i -> [w517]
                                n324 = Concatenate Strings("d" ("string"), w514, "/dt" ("string")) -> (w512:string)
                                n325 = property class="XYGraph"(reference=w518, "Active Plot"=w517, "Plot.Line Width"=u8 2, "Plot.Plot Name"=w512) -> ()  [unwired: 1 in, 2 out]
                                }
                                n326 = property class="XYGraph"(reference=w503, "ScaleLegendVis"=FALSE ("Scale Legend:Visible"), "YScale.NameLbl.Text"="Concentration" ("Label.Text"), "Label.Visible"=FALSE, "Label.FontBold"=TRUE ("Label.Font:Bold"), "LegAutosize"=TRUE ("Legend:Autosize"), "LegPos"=T1 {"Left"=1153, "Top"=25} ("Legend:Position"), "LegNumRows"=w505, "Top"=0 ("Position:Top")) -> ()  [unwired: 1 in, 2 out]
                              }
                            }
                          }
                          frame Enabled {
                          }
                        }
                      }
                    }
                  }
                }
              }
              frame Disabled {
              }
            }
          }
          event Menu Selection (User) {
            n327 = event-data() -> ("ItemTag"=w522:string)  [unwired: 1 in, 6 out]
            n328 = case shown="\"Exit\"" w522 {
              tunnel: [_ _ TRUE ("NewVal") _] -> w521
              tunnel: [w523 w524 w525 w531] -> w520
              tunnel: w519 -> [w523 w524 w525 w530]
              frame "False", Default {
              }
              frame "About D-VASim" {
                n329 = call "About D-VASim.vi"() -> ()  [unwired: 12 in]
              }
              frame "Exit" {
              }
              frame "Open VI" {
                n330 = call "File Dialog"("error in"=w530) -> ("selected path"=w527:path, "cancelled"=w528:bool, "error out"=w529:errorcluster)  [unwired: 11 in, 1 out]
                n331 = case shown="False" w528 {
                  tunnel: [w540 _] -> w531
                  tunnel: w527 -> [w539 _]
                  tunnel: w529 -> [w538 _]
                  frame False {
                    w532 = T10."Standard" ("State")
                    n332 = Open VI Reference(vi path=w539, error in (no error)=w538) -> (vi reference=w537:refnum<vi>, error out=w543:errorcluster)  [unwired: 4 in]
                    n333 = property class="VI"(reference=w537, error in=w543) -> (reference out=w534:refnum<vi>, error out=w533:errorcluster, "FP.State"=w536:T10)
                    n334 = Equal?(x=w536, y=w532) -> (x = y?=w535:bool)
                    n335 = case shown="True" w535 {
                      tunnel: w534 -> [w548 w553]
                      tunnel: [w551 w552] -> w541
                      tunnel: [w549 w553] -> w542
                      tunnel: w533 -> [w546 w552]
                      tunnel: w532 -> [w544 _]
                      frame False {
                        n336 = invoke class="VI" method="FP.Open"(reference=w548, error in=w546, "State"=w544) -> (reference out=w547:refnum<vi>, error out=w545:errorcluster)  [unwired: 2 in, 3 out]
                        n337 = invoke class="VI" method="Run VI"(reference=w547, error in=w545, "Wait until done"=FALSE ("Wait Until Done")) -> (reference out=w549:refnum<vi>, error out=w551:errorcluster)  [unwired: 2 in, 3 out]
                      }
                      frame True {
                      }
                    }
                    n338 = Close Reference(reference=w542, error in (no error)=w541) -> (error out=w540:errorcluster)
                  }
                  frame True {
                  }
                }
              }
            }
          }
          event "Generate SSA VI": Value Change {
            n339 = event-data() -> ("NewVal"=w556:bool)  [unwired: 1 in, 5 out]
            n340 = case shown="True" w556 {
              tunnel: w555 -> [w557 w559]
              tunnel: [w557 w558] -> w554
              frame False {
              }
              frame True {
                n341 = stacked-sequence {
                  seq-local: [w560 _ _ _ _] -> [_ w586 w615 _ _]
                  seq-local: [_ _ _ w619 _] -> [_ _ _ _ w641]
                  seq-local: [_ w585 _ _ _] -> [_ _ _ w618 _]
                  tunnel: w559 -> [w561 _ _ _ _]
                  tunnel: [_ _ _ _ w641] -> w558
                  frame #0 {
                    n342 = disable-structure shown="Disabled" {
                      disable-tunnel: w561 -> [w577 w584]
                      disable-tunnel: [w576 w584] -> w560
                      frame Disabled {
                        n343 = call <vilib>:"Application Directory.vi"() -> ("Application Directory"=w565:path)
                        n344 = Path To String(path=w565) -> (string=w564:string)
                        n345 = Concatenate Strings(w564, ":Sim_Results") -> (w563:string)
                        n346 = local read "Model Name"() -> (w569:string)
                        n347 = String To Path(string=w563) -> (path=w562:path)
                        n348 = Path To String(path=w562) -> (string=w571:string)
                        n349 = List Folder(path=w562, error in=w577) -> (folder names=w574:string[], error out=w568:errorcluster)  [unwired: 2 in, 2 out]
                        n350 = Search 1D Array(1D array=w574, element=w569) -> (index of element=w575:i32)  [unwired: 1 in]
                        n351 = Concatenate Strings(w571, ":", w569) -> (w572:string)
                        n352 = String To Path(string=w572) -> (path=w573:path)
                        n353 = case shown="0, Default" w575 {
                          tunnel: [w579 w583] -> w567
                          tunnel: w573 -> [w579 w582]
                          tunnel: w568 -> [w578 w581]
                          tunnel: [w578 w580] -> w576
                          frame 0, Default {
                          }
                          frame -1 {
                            n354 = Create Folder(path (use dialog)=w582, error in=w581) -> (created path=w583:path, error out=w580:errorcluster)  [unwired: 1 in, 1 out]
                          }
                        }
                        "Model Folder" <- w567
                      }
                      frame Enabled {
                      }
                    }
                  }
                  frame #1 {
                    n355 = disable-structure shown="Enabled" {
                      disable-tunnel: w586 -> [_ w599]
                      disable-tunnel: [_ w598] -> w585
                      frame Disabled {
                        n356 = local read "Model Name"() -> (w591:string)
                        n357 = local read "Model Name"() -> (w592:string)
                        n358 = Concatenate Strings(w591, "_SSA" ("string"), ".vi" ("string")) -> (w588:string)
                        n359 = Concatenate Strings("cp Sub\\ VIs/SSA\\ Template.vi Simulations/" ("command line"), w592, "/" ("string"), w588) -> (w594:string)
                        n360 = call <vilib>:"Application Directory.vi"() -> ("Application Directory"=w587:path)
                        n361 = call <vilib>:"System Exec.vi"("working directory"=w587, "command line"=w594) -> ()  [unwired: 6 in, 4 out]
                      }
                      frame Enabled {
                        n362 = local read "Model Name"() -> (w603:string)
                        n363 = Concatenate Strings(w603, "_SSA" ("string"), ".vi" ("string")) -> (w597:string)
                        "SSA VI Name" <- w597
                        n364 = Concatenate Strings("cmd /c COPY Sim_Results\\SubVIs\\SSA_Template.vi Sim_Results\\" ("command line"), w597) -> (w604:string)
                        n365 = call <vilib>:"Application Directory.vi"() -> ("Application Directory"=w600:path)
                        n366 = call <vilib>:"System Exec.vi"("run minimized? (F)"=TRUE, "error in (no error)"=w599, "working directory"=w600, "command line"=w604) -> ("error out"=w598:errorcluster)  [unwired: 4 in, 3 out]
                      }
                    }
                  }
                  frame #2 {
                    n367 = property class="App"() -> ("App.Kind"=w608:T13)  [unwired: 2 in, 2 out]
                    n368 = case shown="\"Run Time System\"" w608 {
                      tunnel: [_ "cmd /c COPY SBMLComponents.txt Sim_Results\\" ("command line") "cmd /c COPY SBMLComponents.txt Sim_Results\\" ("command line")] -> w607
                      frame "invalid app kind", Default {
                      }
                      frame "Development System" {
                      }
                      frame "Run Time System" {
                      }
                    }
                    n369 = local read "Model Name"() -> (w613:string)
                    n370 = Concatenate Strings(w613, "_SSA" ("string"), ".txt" ("string")) -> (w609:string)
                    "SSA FileName" <- w609
                    n371 = Concatenate Strings(w607, w609) -> (w614:string)
                    n372 = call <vilib>:"Application Directory.vi"() -> ("Application Directory"=w610:path)
                    n373 = call <vilib>:"System Exec.vi"("run minimized? (F)"=TRUE, "error in (no error)"=w615, "working directory"=w610, "command line"=w614) -> ()  [unwired: 4 in, 4 out]
                  }
                  frame #3 {
                    n374 = disable-structure shown="Enabled" {
                      disable-tunnel: [w621 _] -> w619
                      disable-tunnel: w618 -> [w625 _]
                      frame Enabled {
                        n375 = disable-structure shown="Enabled" {
                          disable-tunnel: [w630 w635] -> w627
                          frame Disabled {
                            n376 = local read "Model Folder"() -> (w631:path)
                            n377 = local read "SSA VI Name"() -> (w629:string)
                            n378 = Path To String(path=w631) -> (string=w633:string)
                            n379 = Concatenate Strings(w633, ":", w629) -> (w632:string)
                            n380 = String To Path(string=w632) -> (path=w630:path)
                          }
                          frame Enabled {
                            n381 = local read "SSA VI Name"() -> (w636:string)
                            n382 = call <vilib>:"Application Directory.vi"() -> ("Application Directory"=w637:path)
                            n383 = Path To String(path=w637) -> (string=w639:string)
                            n384 = Concatenate Strings(w639, T9 "\\Sim_Results\\", w636) -> (w640:string)
                            n385 = String To Path(string=w640) -> (path=w635:path)
                          }
                        }
                        n386 = Open VI Reference(vi path=w627, error in (no error)=w625) -> (vi reference=w624:refnum<vi>, error out=w626:errorcluster)  [unwired: 4 in]
                        n387 = invoke class="VI" method="FP.Open"(reference=w624, error in=w626, "State"=T10."Standard") -> (reference out=w623:refnum<vi>, error out=w622:errorcluster)  [unwired: 2 in, 3 out]
                        n388 = invoke class="VI" method="Run VI"(reference=w623, error in=w622, "Wait until done"=FALSE ("Wait Until Done")) -> (error out=w621:errorcluster)  [unwired: 2 in, 4 out]
                      }
                      frame Disabled {
                      }
                    }
                  }
                  frame #4 {
                  }
                }
              }
            }
          }
          event Panel Close? {
            n389 = event-data() -> ()  [unwired: 1 in, 4 out]
            n390 = event-data() -> ()  [unwired: 2 in, 1 out]
          }
        }
      }
    }
  }
  n391 = Current VI's Menubar() -> (w9:refnum<k9>)
  n392 = Delete Menu Items(9:w9) -> (3:w8:refnum<k9>)  [unwired: 3 in, 1 out]
  n393 = Insert Menu Items(7:string[] ["File", "Help"], 9:w8) -> (3:w6:refnum<k9>)  [unwired: 4 in, 2 out]
  n394 = Insert Menu Items(5:"File" ("menu tag"), 7:string[] ["Open VI", "Exit"], 9:w6) -> (3:w1:refnum<k9>)  [unwired: 3 in, 2 out]
  n395 = Insert Menu Items(5:"Help" ("menu tag"), 7:string[] ["About D-VASim"] ("item tags"), 9:w1) -> ()  [unwired: 3 in, 3 out]
  n396 = property class="App"(error in=w11) -> (error out=w10:errorcluster, "App.Kind"=w13:T13)  [unwired: 1 in, 1 out]
  n397 = call <vilib>:"Simple Error Handler.vi"("type of dialog (OK msg:1)"=w12, "error in (no error)"=w10) -> ()  [unwired: 3 in, 5 out]
  n398 = case shown="\"Run Time System\"" w13 {
    frame "invalid app kind", Default {
    }
    frame "Development System" {
    }
    frame "Run Time System" {
      n399 = control-ref of="This VI"() -> (w643:refnum<vi>)
      n400 = invoke class="VI" method="FP.Close"(reference=w643) -> ()  [unwired: 2 in, 3 out]
    }
  }
